vi "BinanceAPI_klinesParser.vi"(0 "String":string="[[1658347200000,\"23663.24000000\",\"23722.59000000\",\"23653.28000000\",\"23714.96000000\",\"256.13989000\",1658347379999,\"6067027.54690940\",9053,\"142.99676000\",\"3387101.46249020\",\"0\"],[1658347380000,\"23718.37000000\",\"23767.73000000\",\"23515.33000000\",\"23543.35000000\",\"946.67772000\",1658347559999,\"22402928.80379690\",22366,\"437.43972000\",\"10355818.28285050\",\"0\"],[1658347560000,\"23543.35000000\",\"23557.69000000\",\"23129.30000000\",\"23290.21000000\",\"3099.94602000\",1658347739999,\"72352782.71562150\",52417,\"1329.12545000\",\"30987661.71943290\",\"0\"],[1658347740000,\"23292.66000000\",\"23362.26000000\",\"23183.57000000\",\"23189.10000000\",\"1104.93990000\",1658347919999,\"25699483.56583190\",26655,\"548.60052000\",\"12760620.12435820\",\"0\"],[1658347920000,\"23186.61000000\",\"23227.93000000\",\"23080.00000000\",\"23085.06000000\",\"1535.74271000\",1658348099999,\"35542160.24309620\",31006,\"720.31062000\",\"16676896.47782450\",\"0\"],[1658348100000,\"23085.06000000\",\"23205.87000000\",\"23061.82000000\",\"23081.44000000\",\"1247.70886000\",1658348279999,\"28838715.14705330\",28358,\"589.19252000\",\"13619917.45208160\",\"0\"],[1658348280000,\"23081.44000000\",\"23146.70000000\",\"23002.89000000\",\"23124.56000000\",\"1176.89567000\",1658348459999,\"27140887.15973450\",27163,\"620.70218000\",\"14315259.40428540\",\"0\"],[1658348460000,\"23128.04000000\",\"23164.75000000\",\"22906.19000000\",\"23077.30000000\",\"2165.26684000\",1658348639999,\"49834566.81714380\",37258,\"1123.79793000\",\"25866736.24309830\",\"0\"],[1658348640000,\"23077.30000000\",\"23266.21000000\",\"23069.87000000\",\"23151.19000000\",\"1420.90968000\",1658348819999,\"32903334.24962870\",30888,\"652.00960000\",\"15098327.30678220\",\"0\"],[1658348820000,\"23154.51000000\",\"23193.68000000\",\"23000.61000000\",\"23030.72000000\",\"870.91964000\",1658348999999,\"20119457.31160460\",22367,\"423.83386000\",\"9792985.11733570\",\"0\"],[1658349000000,\"23030.28000000\",\"23123.57000000\",\"22969.29000000\",\"23104.71000000\",\"1005.49828000\",1658349179999,\"23177047.55477860\",22845,\"498.99542000\",\"11504775.92107370\",\"0\"],[1658349180000,\"23104.71000000\",\"23147.13000000\",\"23031.50000000\",\"23095.39000000\",\"536.59327000\",1658349359999,\"12392897.73165490\",14572,\"241.49870000\",\"5577724.99435290\",\"0\"],[1658349360000,\"23093.23000000\",\"23106.21000000\",\"23018.21000000\",\"23028.14000000\",\"458.30424000\",1658349539999,\"10572885.20125990\",12174,\"216.11603000\",\"4986224.12266900\",\"0\"],[1658349540000,\"23025.72000000\",\"23180.00000000\",\"23010.77000000\",\"23169.63000000\",\"730.04369000\",1658349719999,\"16865565.81021020\",17344,\"391.09889000\",\"9037203.89897580\",\"0\"],[1658349720000,\"23169.63000000\",\"23202.29000000\",\"23104.83000000\",\"23190.76000000\",\"518.70246000\",1658349899999,\"12018650.49457500\",14582,\"284.89408000\",\"6601983.75458750\",\"0\"],[1658349900000,\"23187.58000000\",\"23197.98000000\",\"23117.24000000\",\"23192.65000000\",\"423.00370000\",1658350079999,\"9793254.17683990\",12212,\"207.37017000\",\"4801293.50123250\",\"0\"],[1658350080000,\"23192.65000000\",\"23369.81000000\",\"23188.59000000\",\"23351.47000000\",\"1290.82207000\",1658350259999,\"30067083.65432220\",27695,\"723.29769000\",\"16848129.29270580\",\"0\"],[1658350260000,\"23351.47000000\",\"23370.00000000\",\"23301.63000000\",\"23329.33000000\",\"545.87360000\",1658350439999,\"12735271.72257250\",14658,\"273.13977000\",\"6373064.42542620\",\"0\"],[1658350440000,\"23325.07000000\",\"23348.17000000\",\"23246.78000000\",\"23290.83000000\",\"656.82732000\",1658350619999,\"15299488.59141300\",16542,\"316.26851000\",\"7366633.62180150\",\"0\"],[1658350620000,\"23286.79000000\",\"23315.69000000\",\"23219.44000000\",\"23259.70000000\",\"580.13747000\",1658350799999,\"13504072.32121060\",12670,\"227.22525000\",\"5291058.52408740\",\"0\"],[1658350800000,\"23262.32000000\",\"23307.25000000\",\"23252.06000000\",\"23273.16000000\",\"445.89775000\",1658350979999,\"10382095.07301540\",11907,\"237.41438000\",\"5527766.31736060\",\"0\"],[1658350980000,\"23273.16000000\",\"23317.35000000\",\"23238.07000000\",\"23292.57000000\",\"323.09746000\",1658351159999,\"7522267.57929260\",10583,\"164.20677000\",\"3823461.94073280\",\"0\"],[1658351160000,\"23295.15000000\",\"23408.75000000\",\"23290.50000000\",\"23403.41000000\",\"416.53763000\",1658351339999,\"9730537.88850020\",12557,\"246.43581000\",\"5757447.08477900\",\"0\"],[1658351340000,\"23400.59000000\",\"23404.35000000\",\"23347.74000000\",\"23350.85000000\",\"284.65292000\",1658351519999,\"6651358.99879110\",9465,\"156.28050000\",\"3651802.20196910\",\"0\"],[1658351520000,\"23350.85000000\",\"23388.66000000\",\"23306.08000000\",\"23380.89000000\",\"332.33084000\",1658351699999,\"7759502.79393790\",10066,\"164.48672000\",\"3840378.70951610\",\"0\"],[1658351700000,\"23383.71000000\",\"23389.00000000\",\"23322.20000000\",\"23330.09000000\",\"244.35332000\",1658351879999,\"5706758.02910410\",7878,\"114.35270000\",\"2670918.94295160\",\"0\"],[1658351880000,\"23330.09000000\",\"23382.27000000\",\"23326.32000000\",\"23378.93000000\",\"369.49055000\",1658352059999,\"8631353.96538760\",6569,\"114.80699000\",\"2681833.11026080\",\"0\"],[1658352060000,\"23380.36000000\",\"23434.00000000\",\"23340.00000000\",\"23372.76000000\",\"390.02511000\",1658352239999,\"9122737.93836740\",9832,\"194.24542000\",\"4543845.70816940\",\"0\"],[1658352240000,\"23372.76000000\",\"23372.77000000\",\"23287.28000000\",\"23312.51000000\",\"298.85056000\",1658352419999,\"6973644.48613640\",9193,\"144.27810000\",\"3367082.39989170\",\"0\"],[1658352420000,\"23312.51000000\",\"23345.51000000\",\"23299.38000000\",\"23340.11000000\",\"168.64549000\",1658352599999,\"3932176.69589520\",6031,\"97.74182000\",\"2279375.75222460\",\"0\"],[1658352600000,\"23340.11000000\",\"23347.26000000\",\"23266.42000000\",\"23295.75000000\",\"169.94898000\",1658352779999,\"3958141.00030790\",6143,\"71.57080000\",\"1666862.00138690\",\"0\"],[1658352780000,\"23297.61000000\",\"23350.00000000\",\"23277.48000000\",\"23347.10000000\",\"128.95247000\",1658352959999,\"3005102.45726760\",6498,\"70.34855000\",\"1639681.70112670\",\"0\"],[1658352960000,\"23347.60000000\",\"23379.99000000\",\"23343.23000000\",\"23345.48000000\",\"119.56860000\",1658353139999,\"2793086.41307330\",5469,\"65.88758000\",\"1539242.14634960\",\"0\"],[1658353140000,\"23345.48000000\",\"23347.41000000\",\"23319.58000000\",\"23334.83000000\",\"112.94594000\",1658353319999,\"2635310.06600650\",3781,\"70.77757000\",\"1651431.45277890\",\"0\"],[1658353320000,\"23334.83000000\",\"23700.00000000\",\"23334.83000000\",\"23665.41000000\",\"978.56393000\",1658353499999,\"23032794.93002870\",27892,\"584.67607000\",\"13755496.34479560\",\"0\"],[1658353500000,\"23665.41000000\",\"23799.62000000\",\"23581.75000000\",\"23768.58000000\",\"894.37276000\",1658353679999,\"21213256.93729260\",26896,\"441.60675000\",\"10477754.50332260\",\"0\"],[1658353680000,\"23768.58000000\",\"23769.61000000\",\"23574.81000000\",\"23725.45000000\",\"537.20727000\",1658353859999,\"12724890.73371940\",17629,\"289.57177000\",\"6860726.29343110\",\"0\"],[1658353860000,\"23725.45000000\",\"23733.39000000\",\"23648.88000000\",\"23665.25000000\",\"279.74513000\",1658354039999,\"6625353.22561640\",10688,\"117.34940000\",\"2779141.80989370\",\"0\"],[1658354040000,\"23665.78000000\",\"23686.37000000\",\"23623.54000000\",\"23643.00000000\",\"216.30745000\",1658354219999,\"5116543.37437430\",7874,\"101.28639000\",\"2395812.26952260\",\"0\"],[1658354220000,\"23643.57000000\",\"23652.78000000\",\"23584.36000000\",\"23608.15000000\",\"225.59837000\",1658354399999,\"5327858.79167780\",8462,\"84.56632000\",\"1997358.21979660\",\"0\"],[1658354400000,\"23607.06000000\",\"23616.03000000\",\"23526.38000000\",\"23563.66000000\",\"241.23563000\",1658354579999,\"5686089.41069430\",9460,\"116.03341000\",\"2735055.26742810\",\"0\"],[1658354580000,\"23563.66000000\",\"23641.78000000\",\"23530.04000000\",\"23591.30000000\",\"296.26889000\",1658354759999,\"6984079.86770860\",11005,\"155.97288000\",\"3676126.58231920\",\"0\"],[1658354760000,\"23591.30000000\",\"23635.05000000\",\"23570.20000000\",\"23600.29000000\",\"362.57920000\",1658354939999,\"8556514.96142100\",8070,\"279.40202000\",\"6593791.82218180\",\"0\"],[1658354940000,\"23601.05000000\",\"23601.13000000\",\"23550.00000000\",\"23558.75000000\",\"151.77531000\",1658355119999,\"3577751.06744300\",6127,\"67.94480000\",\"1601722.42267410\",\"0\"],[1658355120000,\"23557.75000000\",\"23579.22000000\",\"23475.00000000\",\"23485.09000000\",\"319.12747000\",1658355299999,\"7508488.55289070\",9656,\"113.02180000\",\"2659377.18639480\",\"0\"],[1658355300000,\"23486.61000000\",\"23544.30000000\",\"23438.76000000\",\"23532.51000000\",\"283.28390000\",1658355479999,\"6657018.16396230\",9873,\"157.38094000\",\"3698445.14656630\",\"0\"],[1658355480000,\"23532.51000000\",\"23538.92000000\",\"23485.02000000\",\"23526.25000000\",\"136.63635000\",1658355659999,\"3213734.04655520\",5849,\"67.83475000\",\"1595511.29869110\",\"0\"],[1658355660000,\"23525.46000000\",\"23581.51000000\",\"23523.52000000\",\"23575.73000000\",\"122.31247000\",1658355839999,\"2879548.45942340\",5190,\"78.42627000\",\"1846524.61665180\",\"0\"],[1658355840000,\"23573.40000000\",\"23584.32000000\",\"23535.77000000\",\"23537.14000000\",\"129.93788000\",1658356019999,\"3060488.05244040\",5764,\"68.74444000\",\"1619190.30047840\",\"0\"],[1658356020000,\"23537.14000000\",\"23550.00000000\",\"23495.01000000\",\"23532.31000000\",\"136.98964000\",1658356199999,\"3223035.76130240\",5999,\"61.78384000\",\"1453672.06304110\",\"0\"],[1658356200000,\"23532.31000000\",\"23574.10000000\",\"23531.00000000\",\"23532.76000000\",\"161.63923000\",1658356379999,\"3806461.12547130\",6658,\"82.11191000\",\"1933603.05814690\",\"0\"],[1658356380000,\"23532.76000000\",\"23533.52000000\",\"23412.99000000\",\"23469.88000000\",\"347.54851000\",1658356559999,\"8158857.45357220\",12563,\"149.67198000\",\"3513318.48321890\",\"0\"],[1658356560000,\"23468.16000000\",\"23492.70000000\",\"23355.00000000\",\"23449.50000000\",\"500.91394000\",1658356739999,\"11738707.50836680\",17277,\"224.26819000\",\"5256198.16761950\",\"0\"],[1658356740000,\"23449.50000000\",\"23460.02000000\",\"23383.93000000\",\"23417.79000000\",\"339.57720000\",1658356919999,\"7953168.25257930\",11805,\"156.70096000\",\"3670040.32626850\",\"0\"],[1658356920000,\"23417.79000000\",\"23445.23000000\",\"23401.59000000\",\"23430.62000000\",\"267.51977000\",1658357099999,\"6266283.00305560\",9666,\"140.04211000\",\"3280368.60094800\",\"0\"],[1658357100000,\"23429.11000000\",\"23430.62000000\",\"23360.00000000\",\"23370.05000000\",\"265.61983000\",1658357279999,\"6215299.54653220\",9837,\"111.43058000\",\"2607569.00195110\",\"0\"],[1658357280000,\"23367.17000000\",\"23410.00000000\",\"23353.04000000\",\"23358.65000000\",\"254.61880000\",1658357459999,\"5953358.79055690\",9842,\"118.64396000\",\"2774327.67614840\",\"0\"],[1658357460000,\"23358.65000000\",\"23376.13000000\",\"23310.43000000\",\"23314.33000000\",\"347.78864000\",1658357639999,\"8118965.53186380\",11790,\"167.28671000\",\"3905541.56132740\",\"0\"],[1658357640000,\"23314.33000000\",\"23367.51000000\",\"23314.33000000\",\"23334.57000000\",\"244.07032000\",1658357819999,\"5696893.81535380\",8896,\"142.33069000\",\"3322310.43938950\",\"0\"],[1658357820000,\"23337.11000000\",\"23357.02000000\",\"23304.56000000\",\"23309.06000000\",\"267.08519000\",1658357999999,\"6230380.52238170\",9247,\"138.65638000\",\"3234636.68335470\",\"0\"],[1658358000000,\"23309.06000000\",\"23334.71000000\",\"23256.69000000\",\"23267.98000000\",\"463.78513000\",1658358179999,\"10806427.81064560\",10604,\"171.91435000\",\"4006041.25282410\",\"0\"],[1658358180000,\"23267.98000000\",\"23280.04000000\",\"23184.25000000\",\"23208.48000000\",\"466.78368000\",1658358359999,\"10840482.69239380\",13918,\"218.86979000\",\"5083327.35367480\",\"0\"],[1658358360000,\"23211.61000000\",\"23300.21000000\",\"23206.00000000\",\"23289.09000000\",\"312.13044000\",1658358539999,\"7259768.03256200\",12194,\"170.57772000\",\"3967277.01586800\",\"0\"],[1658358540000,\"23288.05000000\",\"23317.55000000\",\"23245.00000000\",\"23250.16000000\",\"325.08373000\",1658358719999,\"7565935.03009150\",10181,\"175.10077000\",\"4075930.45346900\",\"0\"],[1658358720000,\"23250.16000000\",\"23265.73000000\",\"23203.57000000\",\"23229.81000000\",\"274.14894000\",1658358899999,\"6367956.05690610\",9199,\"120.91552000\",\"2808717.15305900\",\"0\"],[1658358900000,\"23231.96000000\",\"23264.93000000\",\"23142.57000000\",\"23166.74000000\",\"472.63810000\",1658359079999,\"10962667.84396380\",13410,\"218.02461000\",\"5057754.40926010\",\"0\"],[1658359080000,\"23166.74000000\",\"23231.73000000\",\"23111.00000000\",\"23206.58000000\",\"397.87286000\",1658359259999,\"9221050.64419060\",13655,\"213.01265000\",\"4937189.30769410\",\"0\"],[1658359260000,\"23206.58000000\",\"23268.70000000\",\"23183.30000000\",\"23258.90000000\",\"268.25098000\",1658359439999,\"6230138.32030960\",9875,\"140.72754000\",\"3268798.75356310\",\"0\"],[1658359440000,\"23258.90000000\",\"23287.07000000\",\"23196.00000000\",\"23226.58000000\",\"250.24962000\",1658359619999,\"5815762.30473550\",9116,\"134.23063000\",\"3120068.45655850\",\"0\"],[1658359620000,\"23226.58000000\",\"23244.98000000\",\"23194.14000000\",\"23222.75000000\",\"160.76538000\",1658359799999,\"3732929.12330670\",6448,\"74.87436000\",\"1738725.74384380\",\"0\"],[1658359800000,\"23220.19000000\",\"23251.54000000\",\"23212.84000000\",\"23244.42000000\",\"252.14758000\",1658359979999,\"5858987.19988250\",7956,\"139.04460000\",\"3231264.48457970\",\"0\"],[1658359980000,\"23244.42000000\",\"23357.16000000\",\"23242.73000000\",\"23324.83000000\",\"562.29606000\",1658360159999,\"13110606.53117060\",13800,\"332.75017000\",\"7759117.64943880\",\"0\"],[1658360160000,\"23324.83000000\",\"23347.65000000\",\"23281.71000000\",\"23344.22000000\",\"272.20599000\",1658360339999,\"6345444.66471060\",8282,\"129.69740000\",\"3023748.27259970\",\"0\"],[1658360340000,\"23344.22000000\",\"23391.38000000\",\"23324.61000000\",\"23357.36000000\",\"432.55840000\",1658360519999,\"10101989.86997870\",11211,\"259.52695000\",\"6061286.04227650\",\"0\"],[1658360520000,\"23357.36000000\",\"23396.00000000\",\"23334.43000000\",\"23369.18000000\",\"337.09891000\",1658360699999,\"7877032.48282710\",10322,\"180.01273000\",\"4206442.20913160\",\"0\"],[1658360700000,\"23366.76000000\",\"23401.88000000\",\"23350.00000000\",\"23359.99000000\",\"367.30987000\",1658360879999,\"8586184.09190920\",9435,\"164.34893000\",\"3842234.10386930\",\"0\"],[1658360880000,\"23359.99000000\",\"23378.43000000\",\"23291.13000000\",\"23317.11000000\",\"362.06150000\",1658361059999,\"8450662.03053600\",9310,\"148.28287000\",\"3460709.68962950\",\"0\"],[1658361060000,\"23317.11000000\",\"23326.40000000\",\"23200.44000000\",\"23203.93000000\",\"397.52029000\",1658361239999,\"9257249.64881010\",12151,\"178.48062000\",\"4157326.46055380\",\"0\"],[1658361240000,\"23204.74000000\",\"23268.19000000\",\"23183.10000000\",\"23212.22000000\",\"395.93654000\",1658361419999,\"9194436.55427420\",12573,\"187.68114000\",\"4358614.63933420\",\"0\"],[1658361420000,\"23209.65000000\",\"23241.10000000\",\"23174.67000000\",\"23223.30000000\",\"317.57370000\",1658361599999,\"7370760.20031100\",9690,\"157.06460000\",\"3645875.48688970\",\"0\"],[1658361600000,\"23223.30000000\",\"23280.21000000\",\"23200.00000000\",\"23261.54000000\",\"463.25824000\",1658361779999,\"10767488.43349340\",11878,\"239.67837000\",\"5571170.80147240\",\"0\"],[1658361780000,\"23259.78000000\",\"23314.18000000\",\"23218.01000000\",\"23304.48000000\",\"449.00293000\",1658361959999,\"10453936.81845270\",13318,\"240.94942000\",\"5609923.68490350\",\"0\"],[1658361960000,\"23303.20000000\",\"23317.78000000\",\"23253.39000000\",\"23297.83000000\",\"400.81855000\",1658362139999,\"9337284.98259050\",11991,\"198.82239000\",\"4631841.62327960\",\"0\"],[1658362140000,\"23297.83000000\",\"23315.61000000\",\"23263.93000000\",\"23313.50000000\",\"312.40358000\",1658362319999,\"7275388.40770780\",9482,\"170.74037000\",\"3976401.95753030\",\"0\"],[1658362320000,\"23315.61000000\",\"23350.00000000\",\"23263.66000000\",\"23318.27000000\",\"403.60469000\",1658362499999,\"9406760.13814050\",12022,\"203.22700000\",\"4736873.49560700\",\"0\"],[1658362500000,\"23320.68000000\",\"23386.55000000\",\"23307.91000000\",\"23383.39000000\",\"380.44823000\",1658362679999,\"8883227.63405430\",10580,\"233.56793000\",\"5454053.44543200\",\"0\"],[1658362680000,\"23385.53000000\",\"23386.56000000\",\"23324.21000000\",\"23336.46000000\",\"344.18601000\",1658362859999,\"8038148.69716000\",10173,\"154.85655000\",\"3616470.41552470\",\"0\"],[1658362860000,\"23337.43000000\",\"23339.57000000\",\"23271.40000000\",\"23309.54000000\",\"288.14946000\",1658363039999,\"6714350.49966780\",8922,\"139.56351000\",\"3252097.71397640\",\"0\"],[1658363040000,\"23306.75000000\",\"23334.47000000\",\"23305.02000000\",\"23321.45000000\",\"203.56761000\",1658363219999,\"4746665.90146060\",6832,\"104.78228000\",\"2443295.98027680\",\"0\"],[1658363220000,\"23320.76000000\",\"23348.88000000\",\"23263.24000000\",\"23275.65000000\",\"288.84692000\",1658363399999,\"6731525.37000290\",8880,\"142.81513000\",\"3328246.50960510\",\"0\"],[1658363400000,\"23275.65000000\",\"23282.09000000\",\"23219.72000000\",\"23247.51000000\",\"254.54668000\",1658363579999,\"5918363.44398710\",8334,\"130.64471000\",\"3037435.67776810\",\"0\"],[1658363580000,\"23250.45000000\",\"23254.13000000\",\"23125.00000000\",\"23148.05000000\",\"496.46138000\",1658363759999,\"11505300.14690320\",15124,\"201.66277000\",\"4672724.42245490\",\"0\"],[1658363760000,\"23148.36000000\",\"23221.19000000\",\"23142.00000000\",\"23205.00000000\",\"316.68401000\",1658363939999,\"7342108.47897450\",10074,\"181.63437000\",\"4211144.33656900\",\"0\"],[1658363940000,\"23204.30000000\",\"23206.08000000\",\"23164.95000000\",\"23186.24000000\",\"207.10079000\",1658364119999,\"4801088.55451220\",6923,\"97.75238000\",\"2266153.53402200\",\"0\"],[1658364120000,\"23185.56000000\",\"23200.00000000\",\"23143.15000000\",\"23156.40000000\",\"307.60396000\",1658364299999,\"7126756.39868770\",9282,\"148.03134000\",\"3429901.79666250\",\"0\"],[1658364300000,\"23156.40000000\",\"23191.36000000\",\"23122.34000000\",\"23127.11000000\",\"249.56613000\",1658364479999,\"5780614.14737820\",8355,\"119.76989000\",\"2774269.73107460\",\"0\"],[1658364480000,\"23127.11000000\",\"23175.29000000\",\"23124.65000000\",\"23157.72000000\",\"245.44872000\",1658364659999,\"5682647.90010750\",7937,\"118.12003000\",\"2734724.18187980\",\"0\"],[1658364660000,\"23157.72000000\",\"23211.56000000\",\"23150.02000000\",\"23202.50000000\",\"257.85819000\",1658364839999,\"5977052.10504890\",7840,\"143.23885000\",\"3320381.56935310\",\"0\"],[1658364840000,\"23204.25000000\",\"23267.00000000\",\"23184.43000000\",\"23258.73000000\",\"384.11208000\",1658365019999,\"8920740.54913490\",9756,\"266.40882000\",\"6187599.41639550\",\"0\"],[1658365020000,\"23261.20000000\",\"23276.81000000\",\"23229.28000000\",\"23249.70000000\",\"271.26077000\",1658365199999,\"6307356.11308370\",8670,\"165.52642000\",\"3849099.42916310\",\"0\"],[1658365200000,\"23249.70000000\",\"23312.40000000\",\"23233.07000000\",\"23276.78000000\",\"312.43249000\",1658365379999,\"7271846.46535520\",10029,\"163.17160000\",\"3797986.64275520\",\"0\"],[1658365380000,\"23276.78000000\",\"23302.68000000\",\"23249.67000000\",\"23259.14000000\",\"264.32372000\",1658365559999,\"6152576.59561360\",8370,\"120.86689000\",\"2813668.09538060\",\"0\"],[1658365560000,\"23257.00000000\",\"23294.55000000\",\"23255.42000000\",\"23272.47000000\",\"316.61138000\",1658365739999,\"7368051.92697860\",9505,\"170.44001000\",\"3966369.56429080\",\"0\"],[1658365740000,\"23272.47000000\",\"23289.00000000\",\"23228.95000000\",\"23274.51000000\",\"264.28432000\",1658365919999,\"6148749.23863140\",8936,\"122.00865000\",\"2838814.62197710\",\"0\"],[1658365920000,\"23271.63000000\",\"23442.77000000\",\"23271.63000000\",\"23387.75000000\",\"1133.04116000\",1658366099999,\"26480845.13176050\",27250,\"666.61993000\",\"15579337.89990070\",\"0\"],[1658366100000,\"23389.25000000\",\"23415.84000000\",\"23354.01000000\",\"23364.33000000\",\"372.78877000\",1658366279999,\"8717739.97083280\",12307,\"171.58377000\",\"4012615.56428620\",\"0\"],[1658366280000,\"23364.33000000\",\"23370.53000000\",\"23315.57000000\",\"23344.52000000\",\"304.04739000\",1658366459999,\"7096150.90589430\",10732,\"132.87540000\",\"3101342.08747430\",\"0\"],[1658366460000,\"23346.08000000\",\"23355.90000000\",\"23306.32000000\",\"23336.47000000\",\"260.54737000\",1658366639999,\"6080209.46876510\",8616,\"125.91385000\",\"2938632.88849920\",\"0\"],[1658366640000,\"23336.68000000\",\"23361.22000000\",\"23309.89000000\",\"23313.61000000\",\"206.50235000\",1658366819999,\"4820342.04657080\",7411,\"89.96991000\",\"2100230.98721260\",\"0\"],[1658366820000,\"23313.61000000\",\"23317.89000000\",\"23260.50000000\",\"23261.52000000\",\"275.89735000\",1658366999999,\"6426035.25033980\",9628,\"128.65356000\",\"2996806.27194320\",\"0\"],[1658367000000,\"23261.52000000\",\"23351.21000000\",\"23261.52000000\",\"23345.02000000\",\"345.41077000\",1658367179999,\"8051458.09266070\",9357,\"227.50385000\",\"5302830.05572770\",\"0\"],[1658367180000,\"23343.89000000\",\"23365.16000000\",\"23316.22000000\",\"23317.69000000\",\"223.37271000\",1658367359999,\"5213415.68472510\",7289,\"105.96245000\",\"2473242.49284200\",\"0\"],[1658367360000,\"23317.69000000\",\"23350.39000000\",\"23281.29000000\",\"23340.93000000\",\"308.81026000\",1658367539999,\"7201444.21662230\",7812,\"183.27437000\",\"4273642.49921770\",\"0\"],[1658367540000,\"23340.93000000\",\"23347.81000000\",\"23252.01000000\",\"23287.03000000\",\"297.67650000\",1658367719999,\"6936593.54656370\",9024,\"122.92064000\",\"2864489.34833310\",\"0\"],[1658367720000,\"23285.11000000\",\"23307.04000000\",\"23261.14000000\",\"23297.75000000\",\"176.90967000\",1658367899999,\"4119353.39839250\",6405,\"86.83037000\",\"2021908.85273900\",\"0\"],[1658367900000,\"23299.84000000\",\"23324.00000000\",\"23267.79000000\",\"23285.71000000\",\"227.65603000\",1658368079999,\"5303206.89868370\",7809,\"108.24133000\",\"2521635.12470070\",\"0\"],[1658368080000,\"23287.63000000\",\"23295.72000000\",\"23184.02000000\",\"23208.00000000\",\"520.08759000\",1658368259999,\"12083701.40575020\",12786,\"209.85647000\",\"4876419.35906320\",\"0\"],[1658368260000,\"23208.00000000\",\"23213.15000000\",\"23160.50000000\",\"23185.76000000\",\"350.10841000\",1658368439999,\"8117616.76381720\",11258,\"155.56243000\",\"3606910.48562090\",\"0\"],[1658368440000,\"23183.97000000\",\"23222.36000000\",\"23175.85000000\",\"23192.63000000\",\"217.72169000\",1658368619999,\"5051054.24211660\",6694,\"94.97356000\",\"2203196.80220310\",\"0\"],[1658368620000,\"23194.57000000\",\"23244.73000000\",\"23192.63000000\",\"23235.64000000\",\"180.14749000\",1658368799999,\"4184488.22910970\",5973,\"100.69159000\",\"2338889.82415860\",\"0\"],[1658368800000,\"23233.61000000\",\"23276.51000000\",\"23210.00000000\",\"23275.22000000\",\"201.79844000\",1658368979999,\"4689795.93140160\",6564,\"120.78505000\",\"2807199.10570030\",\"0\"],[1658368980000,\"23275.22000000\",\"23289.96000000\",\"23246.63000000\",\"23284.16000000\",\"245.80435000\",1658369159999,\"5719065.23896820\",8403,\"132.74859000\",\"3088721.22715620\",\"0\"],[1658369160000,\"23285.39000000\",\"23304.83000000\",\"23256.07000000\",\"23260.02000000\",\"210.15150000\",1658369339999,\"4892716.87108830\",7827,\"95.97449000\",\"2234504.66100190\",\"0\"],[1658369340000,\"23260.02000000\",\"23286.52000000\",\"23255.33000000\",\"23272.05000000\",\"152.98457000\",1658369519999,\"3560109.15038380\",6264,\"70.49879000\",\"1640579.52372330\",\"0\"],[1658369520000,\"23271.96000000\",\"23319.73000000\",\"23254.77000000\",\"23303.22000000\",\"177.96559000\",1658369699999,\"4144288.01238590\",7575,\"83.34037000\",\"1940741.68273900\",\"0\"],[1658369700000,\"23302.90000000\",\"23338.51000000\",\"23286.81000000\",\"23297.01000000\",\"214.67452000\",1658369879999,\"5003931.97197020\",8005,\"110.07523000\",\"2565984.71750630\",\"0\"],[1658369880000,\"23298.46000000\",\"23302.39000000\",\"23242.72000000\",\"23253.18000000\",\"200.96737000\",1658370059999,\"4679007.92376780\",7515,\"88.97316000\",\"2071763.38477320\",\"0\"],[1658370060000,\"23253.18000000\",\"23276.15000000\",\"23225.66000000\",\"23231.48000000\",\"178.49990000\",1658370239999,\"4150695.93534270\",7239,\"76.59734000\",\"1781115.64969440\",\"0\"],[1658370240000,\"23230.17000000\",\"23231.52000000\",\"23140.01000000\",\"23145.85000000\",\"561.05378000\",1658370419999,\"13000751.11893660\",15318,\"291.72524000\",\"6759551.68753480\",\"0\"],[1658370420000,\"23145.85000000\",\"23180.34000000\",\"23055.11000000\",\"23085.23000000\",\"650.70228000\",1658370599999,\"15043028.56485940\",15554,\"284.10873000\",\"6568534.39917380\",\"0\"],[1658370600000,\"23088.35000000\",\"23143.09000000\",\"23005.88000000\",\"23137.59000000\",\"888.86232000\",1658370779999,\"20504615.91328710\",20115,\"481.09116000\",\"11098485.83866730\",\"0\"],[1658370780000,\"23136.39000000\",\"23162.51000000\",\"23112.28000000\",\"23125.54000000\",\"286.18338000\",1658370959999,\"6620338.50898710\",8578,\"143.28294000\",\"3314840.00182330\",\"0\"],[1658370960000,\"23125.54000000\",\"23138.92000000\",\"23083.96000000\",\"23086.72000000\",\"210.75822000\",1658371139999,\"4869718.94849060\",7356,\"105.06350000\",\"2427752.43343720\",\"0\"],[1658371140000,\"23084.46000000\",\"23086.73000000\",\"23019.44000000\",\"23066.08000000\",\"591.14488000\",1658371319999,\"13622959.53228690\",16383,\"299.78492000\",\"6908849.76449340\",\"0\"],[1658371320000,\"23064.48000000\",\"23090.60000000\",\"22999.70000000\",\"23001.68000000\",\"668.87831000\",1658371499999,\"15403755.67917970\",14728,\"323.75699000\",\"7456581.31041900\",\"0\"],[1658371500000,\"23003.72000000\",\"23040.00000000\",\"22927.27000000\",\"22934.61000000\",\"959.67221000\",1658371679999,\"22046945.74246740\",22766,\"496.36822000\",\"11405255.13647860\",\"0\"],[1658371680000,\"22934.61000000\",\"22962.02000000\",\"22781.00000000\",\"22876.67000000\",\"1780.19341000\",1658371859999,\"40688265.37866640\",33726,\"730.34572000\",\"16698239.38875990\",\"0\"],[1658371860000,\"22876.67000000\",\"22877.88000000\",\"22809.07000000\",\"22812.90000000\",\"694.37998000\",1658372039999,\"15860142.65244200\",16933,\"358.13122000\",\"8180807.81419470\",\"0\"],[1658372040000,\"22810.08000000\",\"22860.00000000\",\"22714.32000000\",\"22750.41000000\",\"1197.58397000\",1658372219999,\"27271885.70606050\",25860,\"583.33603000\",\"13285722.68335050\",\"0\"],[1658372220000,\"22752.38000000\",\"22788.32000000\",\"22689.42000000\",\"22694.58000000\",\"870.62279000\",1658372399999,\"19784672.42809560\",20446,\"421.41391000\",\"9578329.13338610\",\"0\"],[1658372400000,\"22692.06000000\",\"22751.86000000\",\"22666.00000000\",\"22685.72000000\",\"877.96877000\",1658372579999,\"19937623.63091320\",19760,\"450.54340000\",\"10232467.57196810\",\"0\"],[1658372580000,\"22685.72000000\",\"22801.60000000\",\"22666.00000000\",\"22796.13000000\",\"613.42860000\",1658372759999,\"13957726.91317940\",16984,\"341.18701000\",\"7763524.48165710\",\"0\"],[1658372760000,\"22791.16000000\",\"22818.75000000\",\"22742.92000000\",\"22797.50000000\",\"404.15330000\",1658372939999,\"9207398.19913580\",12824,\"213.56735000\",\"4865813.64813140\",\"0\"],[1658372940000,\"22794.86000000\",\"22842.65000000\",\"22775.26000000\",\"22819.59000000\",\"446.11529000\",1658373119999,\"10178367.01236440\",11873,\"213.59517000\",\"4873371.68049190\",\"0\"],[1658373120000,\"22819.59000000\",\"22833.15000000\",\"22782.04000000\",\"22801.20000000\",\"334.79697000\",1658373299999,\"7635464.97150870\",9139,\"153.88983000\",\"3509856.73091830\",\"0\"],[1658373300000,\"22798.31000000\",\"22830.00000000\",\"22761.75000000\",\"22812.98000000\",\"409.48243000\",1658373479999,\"9338216.08893230\",10253,\"209.64773000\",\"4781706.93003050\",\"0\"],[1658373480000,\"22812.98000000\",\"22866.14000000\",\"22795.15000000\",\"22850.59000000\",\"350.30496000\",1658373659999,\"7999751.47456410\",10593,\"188.12841000\",\"4296239.75612310\",\"0\"],[1658373660000,\"22850.59000000\",\"22862.62000000\",\"22786.28000000\",\"22791.29000000\",\"306.14834000\",1658373839999,\"6985306.34180380\",9205,\"141.03058000\",\"3218032.32110630\",\"0\"],[1658373840000,\"22793.70000000\",\"22805.00000000\",\"22763.50000000\",\"22766.57000000\",\"312.65073000\",1658374019999,\"7124544.77328880\",8236,\"176.33995000\",\"4018827.86364920\",\"0\"],[1658374020000,\"22770.95000000\",\"22791.25000000\",\"22736.45000000\",\"22746.70000000\",\"367.39256000\",1658374199999,\"8363929.17098190\",9444,\"185.67806000\",\"4227495.66403850\",\"0\"],[1658374200000,\"22746.70000000\",\"22767.28000000\",\"22720.37000000\",\"22725.32000000\",\"320.52497000\",1658374379999,\"7291257.83408330\",9253,\"170.21626000\",\"3872145.41741460\",\"0\"],[1658374380000,\"22723.09000000\",\"22815.00000000\",\"22714.56000000\",\"22784.00000000\",\"438.25812000\",1658374559999,\"9979386.59112840\",11004,\"252.88486000\",\"5759396.75949850\",\"0\"],[1658374560000,\"22781.93000000\",\"22861.11000000\",\"22777.80000000\",\"22840.00000000\",\"368.61822000\",1658374739999,\"8414431.74217480\",10221,\"215.28027000\",\"4914252.37777180\",\"0\"],[1658374740000,\"22840.00000000\",\"22855.28000000\",\"22817.44000000\",\"22825.43000000\",\"193.02789000\",1658374919999,\"4407922.17692640\",6435,\"102.74168000\",\"2346405.53148700\",\"0\"],[1658374920000,\"22825.43000000\",\"22830.96000000\",\"22786.42000000\",\"22802.21000000\",\"195.88949000\",1658375099999,\"4467314.49293240\",6597,\"96.84888000\",\"2208671.68410580\",\"0\"],[1658375100000,\"22800.04000000\",\"22853.33000000\",\"22779.12000000\",\"22833.67000000\",\"273.14339000\",1658375279999,\"6231001.97816670\",8210,\"155.36255000\",\"3544333.69735580\",\"0\"],[1658375280000,\"22835.02000000\",\"22850.73000000\",\"22821.26000000\",\"22824.79000000\",\"217.42055000\",1658375459999,\"4964627.09314650\",6869,\"98.18174000\",\"2241989.32999280\",\"0\"],[1658375460000,\"22826.62000000\",\"22841.00000000\",\"22773.45000000\",\"22789.21000000\",\"265.77094000\",1658375639999,\"6061579.92042090\",7287,\"115.53074000\",\"2635091.45940750\",\"0\"],[1658375640000,\"22792.25000000\",\"22839.64000000\",\"22750.50000000\",\"22758.91000000\",\"443.64101000\",1658375819999,\"10110070.99845270\",10403,\"154.01525000\",\"3510513.26605280\",\"0\"],[1658375820000,\"22758.91000000\",\"22796.39000000\",\"22753.92000000\",\"22777.20000000\",\"180.43339000\",1658375999999,\"4109349.84048100\",6581,\"108.06550000\",\"2461206.78180420\",\"0\"],[1658376000000,\"22779.12000000\",\"22860.17000000\",\"22766.00000000\",\"22803.06000000\",\"624.08366000\",1658376179999,\"14242607.74976190\",12668,\"351.77477000\",\"8027617.19641070\",\"0\"],[1658376180000,\"22805.19000000\",\"22812.36000000\",\"22680.39000000\",\"22691.53000000\",\"851.87135000\",1658376359999,\"19381971.86382160\",15110,\"315.41776000\",\"7175318.71990640\",\"0\"],[1658376360000,\"22691.53000000\",\"22750.01000000\",\"22638.53000000\",\"22724.11000000\",\"1008.64261000\",1658376539999,\"22899759.35156330\",20452,\"464.01668000\",\"10534059.20509760\",\"0\"],[1658376540000,\"22723.78000000\",\"22787.50000000\",\"22690.46000000\",\"22751.59000000\",\"470.01808000\",1658376719999,\"10688383.26645950\",11750,\"252.13342000\",\"5733629.75660520\",\"0\"],[1658376720000,\"22751.59000000\",\"22763.17000000\",\"22718.20000000\",\"22755.20000000\",\"341.01248000\",1658376899999,\"7754338.08243520\",8484,\"208.08232000\",\"4731442.48223590\",\"0\"],[1658376900000,\"22750.61000000\",\"22802.41000000\",\"22746.03000000\",\"22794.96000000\",\"408.57760000\",1658377079999,\"9305641.44118390\",11170,\"223.92429000\",\"5100365.62645140\",\"0\"],[1658377080000,\"22794.96000000\",\"22802.77000000\",\"22776.60000000\",\"22794.88000000\",\"294.11685000\",1658377259999,\"6703134.18692500\",7395,\"156.70840000\",\"3571521.76969170\",\"0\"],[1658377260000,\"22794.83000000\",\"22795.56000000\",\"22755.78000000\",\"22756.52000000\",\"204.50335000\",1658377439999,\"4658589.01441900\",6234,\"92.06089000\",\"2097284.34299430\",\"0\"],[1658377440000,\"22760.53000000\",\"22772.69000000\",\"22712.38000000\",\"22733.18000000\",\"281.79796000\",1658377619999,\"6408382.31438280\",7348,\"135.75440000\",\"3087098.72860880\",\"0\"],[1658377620000,\"22733.18000000\",\"22777.04000000\",\"22700.08000000\",\"22732.43000000\",\"301.60760000\",1658377799999,\"6858667.67583850\",8048,\"158.66828000\",\"3608249.98051650\",\"0\"],[1658377800000,\"22734.00000000\",\"22831.08000000\",\"22717.69000000\",\"22814.74000000\",\"644.40953000\",1658377979999,\"14684176.73707260\",14268,\"371.97099000\",\"8476784.16623680\",\"0\"],[1658377980000,\"22814.74000000\",\"22833.35000000\",\"22789.05000000\",\"22822.29000000\",\"299.88180000\",1658378159999,\"6840748.13101670\",8427,\"150.74446000\",\"3439019.88347360\",\"0\"],[1658378160000,\"22823.99000000\",\"22829.17000000\",\"22797.31000000\",\"22822.18000000\",\"179.54466000\",1658378339999,\"4095678.11637340\",5161,\"98.79378000\",\"2253671.73509940\",\"0\"],[1658378340000,\"22822.18000000\",\"22878.00000000\",\"22811.02000000\",\"22840.39000000\",\"443.39911000\",1658378519999,\"10128517.47841070\",9604,\"225.29010000\",\"5146480.56808720\",\"0\"],[1658378520000,\"22840.39000000\",\"22888.00000000\",\"22830.47000000\",\"22858.37000000\",\"417.46955000\",1658378699999,\"9546413.51675720\",7883,\"161.31037000\",\"3688512.76331630\",\"0\"],[1658378700000,\"22858.37000000\",\"22892.89000000\",\"22856.13000000\",\"22888.38000000\",\"251.40187000\",1658378879999,\"5750248.72233290\",6526,\"136.62694000\",\"3125178.12108200\",\"0\"],[1658378880000,\"22888.38000000\",\"22935.20000000\",\"22881.86000000\",\"22918.86000000\",\"502.61385000\",1658379059999,\"11516825.09707570\",11687,\"223.62519000\",\"5124199.85448020\",\"0\"],[1658379060000,\"22917.73000000\",\"22943.18000000\",\"22896.59000000\",\"22896.64000000\",\"300.83256000\",1658379239999,\"6894034.50041330\",7761,\"186.66058000\",\"4277780.57181760\",\"0\"],[1658379240000,\"22899.10000000\",\"22931.50000000\",\"22885.69000000\",\"22912.37000000\",\"170.23739000\",1658379419999,\"3900599.29252590\",5955,\"97.66524000\",\"2237863.88990530\",\"0\"],[1658379420000,\"22912.37000000\",\"22918.95000000\",\"22866.18000000\",\"22881.41000000\",\"286.84166000\",1658379599999,\"6566875.72484430\",7709,\"140.80415000\",\"3223840.33303430\",\"0\"],[1658379600000,\"22881.41000000\",\"22913.10000000\",\"22869.29000000\",\"22899.87000000\",\"179.68967000\",1658379779999,\"4113095.50285550\",5836,\"97.40490000\",\"2229694.80322020\",\"0\"],[1658379780000,\"22899.87000000\",\"22922.00000000\",\"22896.44000000\",\"22917.21000000\",\"171.39995000\",1658379959999,\"3927027.64603680\",6162,\"99.29456000\",\"2275056.38301470\",\"0\"],[1658379960000,\"22917.21000000\",\"22930.43000000\",\"22910.64000000\",\"22929.14000000\",\"142.41097000\",1658380139999,\"3264355.08821520\",5214,\"74.34614000\",\"1704216.77589580\",\"0\"],[1658380140000,\"22929.14000000\",\"22936.67000000\",\"22920.00000000\",\"22931.62000000\",\"193.36071000\",1658380319999,\"4433527.71312080\",5576,\"75.83615000\",\"1738834.21112470\",\"0\"],[1658380320000,\"22931.62000000\",\"22935.32000000\",\"22882.50000000\",\"22903.79000000\",\"184.96537000\",1658380499999,\"4237120.58955230\",5724,\"90.72191000\",\"2078029.56335470\",\"0\"],[1658380500000,\"22903.79000000\",\"22928.04000000\",\"22886.35000000\",\"22917.26000000\",\"140.39499000\",1658380679999,\"3216149.91073640\",5374,\"76.50451000\",\"1752617.07443600\",\"0\"],[1658380680000,\"22918.77000000\",\"22968.46000000\",\"22915.00000000\",\"22943.43000000\",\"314.13101000\",1658380859999,\"7207616.19298830\",7972,\"204.50136000\",\"4692507.46622070\",\"0\"],[1658380860000,\"22943.43000000\",\"22946.09000000\",\"22920.03000000\",\"22931.99000000\",\"131.63220000\",1658381039999,\"3018445.48706260\",5073,\"70.98958000\",\"1627885.70138810\",\"0\"],[1658381040000,\"22929.25000000\",\"22934.46000000\",\"22899.86000000\",\"22906.08000000\",\"248.21723000\",1658381219999,\"5688907.53959740\",5981,\"96.33493000\",\"2207966.97046270\",\"0\"],[1658381220000,\"22903.57000000\",\"22927.03000000\",\"22880.00000000\",\"22885.18000000\",\"188.80546000\",1658381399999,\"4323476.09169620\",5794,\"93.86170000\",\"2149490.81723650\",\"0\"],[1658381400000,\"22885.18000000\",\"22896.28000000\",\"22839.94000000\",\"22847.38000000\",\"256.90405000\",1658381579999,\"5876608.11587860\",7009,\"99.90734000\",\"2285896.98827260\",\"0\"],[1658381580000,\"22847.38000000\",\"22867.23000000\",\"22828.46000000\",\"22855.98000000\",\"223.22515000\",1658381759999,\"5100693.42232280\",6565,\"116.60272000\",\"2664453.46352630\",\"0\"],[1658381760000,\"22857.64000000\",\"22858.18000000\",\"22813.27000000\",\"22845.60000000\",\"367.31704000\",1658381939999,\"8386322.37596330\",9281,\"178.19170000\",\"4068200.14336290\",\"0\"],[1658381940000,\"22842.72000000\",\"22993.71000000\",\"22840.08000000\",\"22951.81000000\",\"726.12788000\",1658382119999,\"16654888.53700440\",17175,\"412.53707000\",\"9461477.84328590\",\"0\"],[1658382120000,\"22951.81000000\",\"22951.81000000\",\"22909.72000000\",\"22918.92000000\",\"248.16104000\",1658382299999,\"5690251.63592150\",6888,\"112.98776000\",\"2590799.45426820\",\"0\"],[1658382300000,\"22918.92000000\",\"22944.30000000\",\"22868.60000000\",\"22893.38000000\",\"266.35280000\",1658382479999,\"6102652.38337950\",7519,\"115.33164000\",\"2642758.03614150\",\"0\"],[1658382480000,\"22896.03000000\",\"22934.36000000\",\"22874.45000000\",\"22925.18000000\",\"314.44447000\",1658382659999,\"7201154.69883880\",8012,\"171.79552000\",\"3934780.01653990\",\"0\"],[1658382660000,\"22922.55000000\",\"22977.07000000\",\"22920.00000000\",\"22954.99000000\",\"328.86120000\",1658382839999,\"7547801.20960840\",8661,\"186.44438000\",\"4279491.51163780\",\"0\"],[1658382840000,\"22954.99000000\",\"22967.31000000\",\"22866.63000000\",\"22909.93000000\",\"536.81207000\",1658383019999,\"12298087.69139920\",12500,\"223.16844000\",\"5112581.66185750\",\"0\"],[1658383020000,\"22907.31000000\",\"22945.63000000\",\"22891.87000000\",\"22942.00000000\",\"227.36534000\",1658383199999,\"5211381.78234630\",7506,\"114.70388000\",\"2629140.41163150\",\"0\"],[1658383200000,\"22943.15000000\",\"22948.65000000\",\"22916.24000000\",\"22922.55000000\",\"209.48163000\",1658383379999,\"4803746.93690640\",5994,\"108.92101000\",\"2497668.21469610\",\"0\"],[1658383380000,\"22920.43000000\",\"22937.78000000\",\"22904.68000000\",\"22924.56000000\",\"163.64493000\",1658383559999,\"3750758.09159140\",5979,\"82.04286000\",\"1880474.35091930\",\"0\"],[1658383560000,\"22926.67000000\",\"22964.67000000\",\"22911.38000000\",\"22946.26000000\",\"374.96605000\",1658383739999,\"8603558.27681430\",9379,\"212.27878000\",\"4870928.00449820\",\"0\"],[1658383740000,\"22946.26000000\",\"22967.57000000\",\"22937.70000000\",\"22942.59000000\",\"212.91666000\",1658383919999,\"4887115.27655360\",6503,\"100.48061000\",\"2306543.09886280\",\"0\"],[1658383920000,\"22940.22000000\",\"22963.24000000\",\"22939.00000000\",\"22953.57000000\",\"222.61792000\",1658384099999,\"5109407.86712630\",6435,\"125.43550000\",\"2879047.82131130\",\"0\"],[1658384100000,\"22953.57000000\",\"22953.57000000\",\"22917.05000000\",\"22923.07000000\",\"190.14514000\",1658384279999,\"4361832.81695020\",6526,\"86.46890000\",\"1983733.60690850\",\"0\"],[1658384280000,\"22923.07000000\",\"22944.37000000\",\"22903.43000000\",\"22928.21000000\",\"180.06834000\",1658384459999,\"4127660.43491110\",6245,\"79.72815000\",\"1827645.17770050\",\"0\"],[1658384460000,\"22931.45000000\",\"22938.72000000\",\"22885.19000000\",\"22908.28000000\",\"311.58441000\",1658384639999,\"7136634.70334500\",7953,\"170.22737000\",\"3898854.94508950\",\"0\"],[1658384640000,\"22905.78000000\",\"22928.91000000\",\"22890.73000000\",\"22915.26000000\",\"271.88054000\",1658384819999,\"6229485.56860730\",7448,\"162.10243000\",\"3714226.15544010\",\"0\"],[1658384820000,\"22916.57000000\",\"22936.83000000\",\"22876.01000000\",\"22882.69000000\",\"224.73649000\",1658384999999,\"5148892.23478750\",7214,\"109.87713000\",\"2518000.53228900\",\"0\"],[1658385000000,\"22882.69000000\",\"22890.00000000\",\"22806.25000000\",\"22826.61000000\",\"456.97170000\",1658385179999,\"10443029.49273590\",11939,\"198.20989000\",\"4529858.73189110\",\"0\"],[1658385180000,\"22829.04000000\",\"22857.36000000\",\"22823.41000000\",\"22842.99000000\",\"178.42730000\",1658385359999,\"4075677.74077730\",7071,\"94.23281000\",\"2152566.03852940\",\"0\"],[1658385360000,\"22840.82000000\",\"22882.37000000\",\"22840.82000000\",\"22864.71000000\",\"225.89921000\",1658385539999,\"5165389.69056830\",7561,\"120.05834000\",\"2745347.58441100\",\"0\"],[1658385540000,\"22864.70000000\",\"22873.92000000\",\"22831.72000000\",\"22863.53000000\",\"170.35168000\",1658385719999,\"3893056.08833230\",6540,\"81.69606000\",\"1866987.71892780\",\"0\"],[1658385720000,\"22863.53000000\",\"22877.58000000\",\"22845.84000000\",\"22857.81000000\",\"152.74665000\",1658385899999,\"3492018.47639480\",5967,\"74.32423000\",\"1699281.46230070\",\"0\"],[1658385900000,\"22857.81000000\",\"22862.83000000\",\"22813.33000000\",\"22819.50000000\",\"195.57316000\",1658386079999,\"4465692.00162510\",6596,\"85.61011000\",\"1954802.86704320\",\"0\"],[1658386080000,\"22819.50000000\",\"22827.08000000\",\"22750.14000000\",\"22804.05000000\",\"711.78081000\",1658386259999,\"16223086.43974410\",14767,\"327.02593000\",\"7454207.90476280\",\"0\"],[1658386260000,\"22798.75000000\",\"22811.70000000\",\"22755.13000000\",\"22801.04000000\",\"336.73897000\",1658386439999,\"7670544.43493360\",9670,\"155.25172000\",\"3536704.74040360\",\"0\"],[1658386440000,\"22803.11000000\",\"22833.14000000\",\"22793.10000000\",\"22822.63000000\",\"268.55820000\",1658386619999,\"6127836.89247470\",7636,\"156.47482000\",\"3570594.22088140\",\"0\"],[1658386620000,\"22822.63000000\",\"22824.85000000\",\"22773.07000000\",\"22790.23000000\",\"177.20604000\",1658386799999,\"4039364.91360110\",6753,\"63.01814000\",\"1436504.62145050\",\"0\"],[1658386800000,\"22790.23000000\",\"22812.05000000\",\"22773.49000000\",\"22812.02000000\",\"199.98118000\",1658386979999,\"4558446.91758840\",7111,\"97.40238000\",\"2220424.13180600\",\"0\"],[1658386980000,\"22812.02000000\",\"22827.27000000\",\"22778.27000000\",\"22796.92000000\",\"245.74473000\",1658387159999,\"5604657.15180260\",7543,\"121.33836000\",\"2767570.84143610\",\"0\"],[1658387160000,\"22796.90000000\",\"22874.27000000\",\"22781.97000000\",\"22865.26000000\",\"384.61423000\",1658387339999,\"8784370.57386480\",10206,\"229.90772000\",\"5251151.73593280\",\"0\"],[1658387340000,\"22865.26000000\",\"22921.12000000\",\"22843.50000000\",\"22904.99000000\",\"432.62601000\",1658387519999,\"9904425.33851090\",12614,\"245.86837000\",\"5628843.48165190\",\"0\"],[1658387520000,\"22904.99000000\",\"22943.94000000\",\"22882.51000000\",\"22912.64000000\",\"647.79025000\",1658387699999,\"14843731.20131320\",11463,\"290.60354000\",\"6659599.90530960\",\"0\"],[1658387700000,\"22912.64000000\",\"22943.21000000\",\"22865.55000000\",\"22941.54000000\",\"420.55435000\",1658387879999,\"9631843.50574210\",9617,\"233.31441000\",\"5343540.28151000\",\"0\"],[1658387880000,\"22936.96000000\",\"23099.51000000\",\"22932.96000000\",\"23057.10000000\",\"1739.25815000\",1658388059999,\"40057271.17942390\",26386,\"741.81748000\",\"17084765.79160620\",\"0\"],[1658388060000,\"23057.10000000\",\"23082.60000000\",\"23047.35000000\",\"23049.03000000\",\"355.88216000\",1658388239999,\"8206660.37207080\",9719,\"167.53008000\",\"3863488.74113670\",\"0\"],[1658388240000,\"23047.36000000\",\"23050.96000000\",\"22955.52000000\",\"23010.00000000\",\"499.60329000\",1658388419999,\"11490645.33288960\",13045,\"233.08045000\",\"5360555.84677680\",\"0\"],[1658388420000,\"23010.00000000\",\"23019.81000000\",\"22983.81000000\",\"22998.08000000\",\"200.72656000\",1658388599999,\"4616885.16137110\",7703,\"102.69488000\",\"2362114.45552810\",\"0\"],[1658388600000,\"22998.08000000\",\"23006.75000000\",\"22956.01000000\",\"22973.79000000\",\"217.33793000\",1658388779999,\"4994168.82331690\",7408,\"111.10109000\",\"2553121.14735140\",\"0\"],[1658388780000,\"22973.79000000\",\"22975.68000000\",\"22940.70000000\",\"22941.03000000\",\"261.64217000\",1658388959999,\"6006671.09483550\",7636,\"96.01176000\",\"2204397.80781890\",\"0\"],[1658388960000,\"22944.12000000\",\"23032.23000000\",\"22928.89000000\",\"23022.21000000\",\"381.25189000\",1658389139999,\"8763041.15805490\",10219,\"202.68765000\",\"4658429.65086230\",\"0\"],[1658389140000,\"23022.21000000\",\"23038.44000000\",\"22980.32000000\",\"22993.68000000\",\"266.72718000\",1658389319999,\"6137314.14042570\",8125,\"120.02034000\",\"2761803.80804330\",\"0\"],[1658389320000,\"22993.69000000\",\"23009.91000000\",\"22966.45000000\",\"22989.99000000\",\"241.70446000\",1658389499999,\"5555191.41622610\",7983,\"114.38061000\",\"2628989.62966860\",\"0\"],[1658389500000,\"22989.99000000\",\"23000.00000000\",\"22973.18000000\",\"22976.65000000\",\"158.39607000\",1658389679999,\"3641235.53285830\",6618,\"74.57911000\",\"1714508.07042070\",\"0\"],[1658389680000,\"22978.75000000\",\"22981.87000000\",\"22938.99000000\",\"22947.42000000\",\"219.12320000\",1658389859999,\"5030866.76187350\",7463,\"102.22774000\",\"2347137.76131960\",\"0\"],[1658389860000,\"22949.51000000\",\"22980.09000000\",\"22920.80000000\",\"22970.73000000\",\"253.56143000\",1658390039999,\"5819190.95566990\",8112,\"130.43720000\",\"2993625.69932110\",\"0\"],[1658390040000,\"22970.73000000\",\"22979.55000000\",\"22955.14000000\",\"22962.05000000\",\"257.47149000\",1658390219999,\"5913804.16505150\",6850,\"121.06409000\",\"2780632.07660740\",\"0\"],[1658390220000,\"22962.05000000\",\"22964.33000000\",\"22919.33000000\",\"22931.56000000\",\"217.43307000\",1658390399999,\"4987771.82405600\",7121,\"98.72213000\",\"2264794.84287690\",\"0\"],[1658390400000,\"22929.28000000\",\"22936.26000000\",\"22880.50000000\",\"22921.29000000\",\"427.53097000\",1658390579999,\"9792635.79032000\",11315,\"188.51373000\",\"4317950.35628020\",\"0\"],[1658390580000,\"22921.29000000\",\"22971.34000000\",\"22910.00000000\",\"22935.80000000\",\"279.66069000\",1658390759999,\"6415552.01937990\",8685,\"154.73621000\",\"3549956.43260070\",\"0\"],[1658390760000,\"22935.80000000\",\"22939.07000000\",\"22900.00000000\",\"22926.48000000\",\"301.24596000\",1658390939999,\"6903706.34004860\",8825,\"147.43593000\",\"3379202.07618100\",\"0\"],[1658390940000,\"22926.48000000\",\"22934.48000000\",\"22910.42000000\",\"22928.89000000\",\"129.96802000\",1658391119999,\"2979205.29757110\",5528,\"66.83450000\",\"1532063.22619490\",\"0\"],[1658391120000,\"22928.90000000\",\"22931.53000000\",\"22872.50000000\",\"22886.16000000\",\"267.39027000\",1658391299999,\"6123609.48497560\",7855,\"113.77128000\",\"2605609.65347740\",\"0\"],[1658391300000,\"22886.16000000\",\"22932.09000000\",\"22863.78000000\",\"22924.16000000\",\"279.66147000\",1658391479999,\"6404613.75773770\",8916,\"153.49100000\",\"3515508.74294250\",\"0\"],[1658391480000,\"22922.19000000\",\"22924.35000000\",\"22850.69000000\",\"22853.60000000\",\"215.96850000\",1658391659999,\"4941549.48785070\",7271,\"91.79903000\",\"2100462.39088830\",\"0\"],[1658391660000,\"22853.60000000\",\"22888.84000000\",\"22837.92000000\",\"22851.63000000\",\"292.77461000\",1658391839999,\"6694424.51584300\",8748,\"142.01439000\",\"3247375.07608080\",\"0\"],[1658391840000,\"22851.63000000\",\"22859.00000000\",\"22815.86000000\",\"22837.55000000\",\"309.40893000\",1658392019999,\"7066768.10339130\",9894,\"155.39354000\",\"3549220.35745520\",\"0\"],[1658392020000,\"22838.72000000\",\"22851.82000000\",\"22820.00000000\",\"22835.28000000\",\"174.51439000\",1658392199999,\"3985382.35038390\",6620,\"88.78070000\",\"2027502.90973130\",\"0\"],[1658392200000,\"22833.56000000\",\"22859.99000000\",\"22820.69000000\",\"22856.91000000\",\"192.83593000\",1658392379999,\"4404868.03625510\",7521,\"100.41024000\",\"2293751.77845230\",\"0\"],[1658392380000,\"22856.91000000\",\"22911.16000000\",\"22851.37000000\",\"22868.92000000\",\"324.03507000\",1658392559999,\"7415448.31160220\",9537,\"178.53841000\",\"4085879.73469440\",\"0\"],[1658392560000,\"22867.24000000\",\"22904.87000000\",\"22863.57000000\",\"22893.04000000\",\"241.48843000\",1658392739999,\"5526402.51428680\",7267,\"128.86156000\",\"2948990.57325590\",\"0\"],[1658392740000,\"22895.25000000\",\"22915.22000000\",\"22836.68000000\",\"22873.35000000\",\"556.71895000\",1658392919999,\"12741179.16748020\",12205,\"321.48285000\",\"7359135.44422970\",\"0\"],[1658392920000,\"22875.80000000\",\"22887.78000000\",\"22825.91000000\",\"22829.94000000\",\"555.99498000\",1658393099999,\"12708125.11815770\",14191,\"281.89757000\",\"6443831.51286480\",\"0\"],[1658393100000,\"22833.37000000\",\"22842.10000000\",\"22797.03000000\",\"22810.73000000\",\"432.04330000\",1658393279999,\"9857324.55330810\",10049,\"227.04479000\",\"5180439.81705170\",\"0\"],[1658393280000,\"22808.69000000\",\"22881.12000000\",\"22800.27000000\",\"22873.77000000\",\"312.45927000\",1658393459999,\"7133303.77650850\",9083,\"204.71151000\",\"4673806.81971470\",\"0\"],[1658393460000,\"22873.45000000\",\"22897.22000000\",\"22842.81000000\",\"22857.82000000\",\"267.54929000\",1658393639999,\"6117809.95680980\",8423,\"138.13486000\",\"3158797.77054820\",\"0\"],[1658393640000,\"22856.28000000\",\"22870.65000000\",\"22844.45000000\",\"22859.55000000\",\"157.54947000\",1658393819999,\"3601280.40439370\",5903,\"91.83657000\",\"2099290.10136510\",\"0\"],[1658393820000,\"22862.30000000\",\"22878.77000000\",\"22851.70000000\",\"22878.77000000\",\"146.64888000\",1658393999999,\"3352970.57750520\",5933,\"75.89196000\",\"1735258.96881760\",\"0\"],[1658394000000,\"22878.77000000\",\"22887.76000000\",\"22866.20000000\",\"22883.54000000\",\"152.31468000\",1658394179999,\"3484506.62602830\",6021,\"75.83327000\",\"1734935.32494880\",\"0\"],[1658394180000,\"22883.54000000\",\"22889.06000000\",\"22855.29000000\",\"22887.27000000\",\"228.85878000\",1658394359999,\"5233703.64289330\",7194,\"115.38850000\",\"2639020.63786090\",\"0\"],[1658394360000,\"22886.79000000\",\"22951.97000000\",\"22884.10000000\",\"22893.30000000\",\"499.62268000\",1658394539999,\"11448770.93012090\",11873,\"298.63996000\",\"6843206.11955470\",\"0\"],[1658394540000,\"22891.35000000\",\"22935.77000000\",\"22891.33000000\",\"22928.55000000\",\"218.25781000\",1658394719999,\"5000495.67707020\",7276,\"118.05086000\",\"2704672.92922560\",\"0\"],[1658394720000,\"22927.40000000\",\"22970.90000000\",\"22916.74000000\",\"22948.39000000\",\"402.35551000\",1658394899999,\"9230663.78449500\",11148,\"204.94155000\",\"4701610.74035630\",\"0\"],[1658394900000,\"22949.66000000\",\"23002.63000000\",\"22943.91000000\",\"22990.57000000\",\"502.21338000\",1658395079999,\"11539081.45203720\",13482,\"257.41829000\",\"5915119.23715040\",\"0\"],[1658395080000,\"22987.48000000\",\"23004.31000000\",\"22964.40000000\",\"22997.24000000\",\"374.15279000\",1658395259999,\"8601305.04050000\",10843,\"204.00695000\",\"4690005.52921410\",\"0\"],[1658395260000,\"22994.94000000\",\"22997.28000000\",\"22930.61000000\",\"22940.46000000\",\"261.57552000\",1658395439999,\"6006450.16647190\",8785,\"109.30566000\",\"2510125.09450610\",\"0\"],[1658395440000,\"22940.46000000\",\"22984.09000000\",\"22916.83000000\",\"22974.95000000\",\"366.11048000\",1658395619999,\"8403427.60175220\",9505,\"184.88870000\",\"4243870.26641410\",\"0\"],[1658395620000,\"22971.76000000\",\"22978.35000000\",\"22935.55000000\",\"22947.37000000\",\"221.41411000\",1658395799999,\"5082528.90967880\",7661,\"103.93921000\",\"2385915.18790580\",\"0\"],[1658395800000,\"22947.37000000\",\"23000.00000000\",\"22934.91000000\",\"22992.48000000\",\"211.43008000\",1658395979999,\"4855278.42314780\",7010,\"126.79597000\",\"2912173.18897860\",\"0\"],[1658395980000,\"22990.95000000\",\"23022.54000000\",\"22945.66000000\",\"22947.25000000\",\"328.36529000\",1658396159999,\"7546839.94344890\",9083,\"171.51209000\",\"3942078.19359990\",\"0\"],[1658396160000,\"22949.61000000\",\"22970.98000000\",\"22942.00000000\",\"22961.32000000\",\"143.57179000\",1658396339999,\"3295516.08117440\",5702,\"83.47467000\",\"1916102.48350980\",\"0\"],[1658396340000,\"22961.32000000\",\"22974.27000000\",\"22924.17000000\",\"22960.58000000\",\"252.86384000\",1658396519999,\"5803525.99576260\",7641,\"119.41055000\",\"2740689.79252690\",\"0\"],[1658396520000,\"22963.46000000\",\"22983.89000000\",\"22945.31000000\",\"22950.70000000\",\"221.04601000\",1658396699999,\"5076082.30296960\",7428,\"105.86488000\",\"2431165.73387100\",\"0\"],[1658396700000,\"22950.70000000\",\"22988.00000000\",\"22944.53000000\",\"22980.77000000\",\"214.31536000\",1658396879999,\"4921547.76552000\",7323,\"118.90269000\",\"2730772.03082620\",\"0\"],[1658396880000,\"22983.53000000\",\"22993.64000000\",\"22940.63000000\",\"22945.62000000\",\"236.55521000\",1658397059999,\"5432924.00784820\",8017,\"111.95963000\",\"2571691.49717520\",\"0\"],[1658397060000,\"22945.62000000\",\"22986.52000000\",\"22928.48000000\",\"22972.28000000\",\"298.47844000\",1658397239999,\"6853351.74839070\",8938,\"179.47309000\",\"4120922.14224560\",\"0\"],[1658397240000,\"22970.11000000\",\"22998.00000000\",\"22958.86000000\",\"22986.30000000\",\"246.73385000\",1658397419999,\"5670591.85571780\",8201,\"125.94080000\",\"2894674.99177830\",\"0\"],[1658397420000,\"22986.30000000\",\"23006.57000000\",\"22971.46000000\",\"23003.58000000\",\"205.86029000\",1658397599999,\"4732907.98005690\",7145,\"125.24913000\",\"2879701.68286560\",\"0\"],[1658397600000,\"23003.58000000\",\"23039.67000000\",\"22979.54000000\",\"23032.52000000\",\"399.34853000\",1658397779999,\"9186461.90802340\",11132,\"240.64782000\",\"5536038.50434450\",\"0\"],[1658397780000,\"23034.26000000\",\"23057.78000000\",\"23005.39000000\",\"23023.34000000\",\"316.96058000\",1658397959999,\"7299589.92089620\",10716,\"175.71287000\",\"4046778.99419850\",\"0\"],[1658397960000,\"23025.60000000\",\"23031.91000000\",\"23002.95000000\",\"23027.49000000\",\"232.17639000\",1658398139999,\"5343852.42254820\",7990,\"110.62503000\",\"2546269.29116590\",\"0\"],[1658398140000,\"23024.59000000\",\"23048.87000000\",\"22996.98000000\",\"23026.53000000\",\"350.87691000\",1658398319999,\"8078056.76425320\",9317,\"141.78906000\",\"3264505.58554490\",\"0\"],[1658398320000,\"23026.54000000\",\"23074.12000000\",\"23019.00000000\",\"23050.27000000\",\"260.36195000\",1658398499999,\"5998875.14884080\",8560,\"143.98826000\",\"3317708.51668410\",\"0\"],[1658398500000,\"23050.27000000\",\"23071.44000000\",\"23008.01000000\",\"23013.57000000\",\"278.31312000\",1658398679999,\"6412434.98167830\",9317,\"142.63446000\",\"3286538.17011550\",\"0\"],[1658398680000,\"23013.57000000\",\"23016.17000000\",\"22972.24000000\",\"23005.04000000\",\"316.86137000\",1658398859999,\"7286940.15762550\",9315,\"173.75114000\",\"3995906.65356120\",\"0\"],[1658398860000,\"23005.04000000\",\"23007.58000000\",\"22974.98000000\",\"22993.41000000\",\"305.31864000\",1658399039999,\"7018576.34409120\",8529,\"141.34760000\",\"3249325.71200520\",\"0\"],[1658399040000,\"22993.41000000\",\"22999.48000000\",\"22966.32000000\",\"22977.85000000\",\"231.80601000\",1658399219999,\"5327001.49873450\",7498,\"95.84516000\",\"2202670.72371250\",\"0\"],[1658399220000,\"22977.85000000\",\"22985.76000000\",\"22958.37000000\",\"22972.31000000\",\"178.20296000\",1658399399999,\"4093841.47361100\",6633,\"87.44139000\",\"2008956.47039280\",\"0\"],[1658399400000,\"22970.34000000\",\"23000.59000000\",\"22958.01000000\",\"22973.49000000\",\"268.10925000\",1658399579999,\"6161946.16535390\",9132,\"128.93400000\",\"2963458.27059010\",\"0\"],[1658399580000,\"22971.69000000\",\"22977.00000000\",\"22937.02000000\",\"22950.84000000\",\"228.20147000\",1658399759999,\"5237842.66226200\",7988,\"115.37167000\",\"2648166.35437760\",\"0\"],[1658399760000,\"22950.84000000\",\"22959.90000000\",\"22937.41000000\",\"22953.28000000\",\"184.15400000\",1658399939999,\"4226081.25687060\",7045,\"94.75421000\",\"2174566.27188540\",\"0\"],[1658399940000,\"22955.00000000\",\"22964.12000000\",\"22931.00000000\",\"22947.19000000\",\"271.76044000\",1658400119999,\"6236145.26080700\",8142,\"145.48737000\",\"3338686.69213890\",\"0\"],[1658400120000,\"22947.19000000\",\"22954.66000000\",\"22935.00000000\",\"22945.87000000\",\"220.00989000\",1658400299999,\"5047614.25447990\",7025,\"155.88410000\",\"3576457.12111180\",\"0\"],[1658400300000,\"22945.87000000\",\"22954.45000000\",\"22935.78000000\",\"22939.96000000\",\"166.28591000\",1658400479999,\"3815242.09580000\",6684,\"92.28674000\",\"2117446.23542700\",\"0\"],[1658400480000,\"22941.63000000\",\"22960.62000000\",\"22923.59000000\",\"22943.63000000\",\"208.85245000\",1658400659999,\"4791443.50315880\",8540,\"108.52271000\",\"2489719.12608130\",\"0\"],[1658400660000,\"22946.87000000\",\"22980.09000000\",\"22943.63000000\",\"22952.72000000\",\"194.65942000\",1658400839999,\"4470091.35245520\",7535,\"113.62805000\",\"2609383.67815740\",\"0\"],[1658400840000,\"22952.72000000\",\"22954.73000000\",\"22885.00000000\",\"22902.38000000\",\"440.25432000\",1658401019999,\"10084490.83086460\",11569,\"189.94875000\",\"4350871.59529620\",\"0\"],[1658401020000,\"22904.29000000\",\"22908.06000000\",\"22846.95000000\",\"22869.55000000\",\"359.42875000\",1658401199999,\"8222398.69070540\",10032,\"182.31364000\",\"4170603.41238790\",\"0\"],[1658401200000,\"22870.88000000\",\"22878.33000000\",\"22827.58000000\",\"22832.19000000\",\"311.53208000\",1658401379999,\"7118412.72356050\",9464,\"152.06684000\",\"3474937.57620450\",\"0\"],[1658401380000,\"22832.19000000\",\"22865.56000000\",\"22817.93000000\",\"22852.60000000\",\"369.88390000\",1658401559999,\"8448846.39341650\",11027,\"201.78029000\",\"4609285.61970110\",\"0\"],[1658401560000,\"22852.60000000\",\"22888.00000000\",\"22844.72000000\",\"22881.37000000\",\"217.73664000\",1658401739999,\"4978640.66978540\",7830,\"129.78175000\",\"2967612.17040220\",\"0\"],[1658401740000,\"22881.37000000\",\"22906.87000000\",\"22850.63000000\",\"22850.63000000\",\"302.81163000\",1658401919999,\"6929118.61308830\",8806,\"145.34593000\",\"3326500.99181780\",\"0\"],[1658401920000,\"22853.61000000\",\"22853.62000000\",\"22662.65000000\",\"22699.53000000\",\"1046.41872000\",1658402099999,\"23822679.26519460\",20970,\"395.48112000\",\"9002703.85722050\",\"0\"],[1658402100000,\"22698.21000000\",\"22740.00000000\",\"22650.00000000\",\"22716.47000000\",\"860.01313000\",1658402279999,\"19519878.53062770\",21303,\"460.84065000\",\"10461840.19543610\",\"0\"],[1658402280000,\"22718.42000000\",\"22778.90000000\",\"22708.04000000\",\"22724.75000000\",\"703.91157000\",1658402459999,\"16009241.59192930\",14252,\"431.45165000\",\"9813188.07878430\",\"0\"],[1658402460000,\"22722.03000000\",\"22795.00000000\",\"22722.03000000\",\"22746.10000000\",\"476.50023000\",1658402639999,\"10843738.75501340\",10497,\"285.83867000\",\"6505353.96856580\",\"0\"],[1658402640000,\"22742.85000000\",\"22748.58000000\",\"22692.62000000\",\"22708.75000000\",\"450.22786000\",1658402819999,\"10227580.72239830\",10140,\"245.28853000\",\"5571985.15440420\",\"0\"],[1658402820000,\"22708.91000000\",\"22730.62000000\",\"22466.34000000\",\"22562.44000000\",\"1976.24407000\",1658402999999,\"44583666.16286020\",34168,\"856.17116000\",\"19311062.30014440\",\"0\"],[1658403000000,\"22562.44000000\",\"22637.26000000\",\"22536.34000000\",\"22597.25000000\",\"868.43448000\",1658403179999,\"19622764.45435830\",18482,\"467.79452000\",\"10569862.96765350\",\"0\"],[1658403180000,\"22594.52000000\",\"22647.74000000\",\"22570.14000000\",\"22632.26000000\",\"1194.97140000\",1658403359999,\"27011441.13157010\",21445,\"810.34086000\",\"18316918.09918060\",\"0\"],[1658403360000,\"22633.74000000\",\"22636.69000000\",\"22555.57000000\",\"22593.70000000\",\"705.06683000\",1658403539999,\"15925659.39825940\",16742,\"358.19987000\",\"8091310.93737440\",\"0\"],[1658403540000,\"22593.50000000\",\"22598.86000000\",\"22540.65000000\",\"22554.47000000\",\"512.40950000\",1658403719999,\"11562297.22239780\",13948,\"256.05004000\",\"5778032.22542090\",\"0\"],[1658403720000,\"22554.47000000\",\"22611.99000000\",\"22551.24000000\",\"22606.38000000\",\"456.56067000\",1658403899999,\"10312507.04765190\",12420,\"259.53849000\",\"5862714.99864330\",\"0\"],[1658403900000,\"22609.62000000\",\"22664.03000000\",\"22590.02000000\",\"22625.69000000\",\"579.11977000\",1658404079999,\"13106692.85888270\",11796,\"303.91456000\",\"6878854.41662260\",\"0\"],[1658404080000,\"22623.97000000\",\"22663.64000000\",\"22617.00000000\",\"22657.13000000\",\"378.06206000\",1658404259999,\"8562473.84216890\",8461,\"169.43015000\",\"3837433.83433870\",\"0\"],[1658404260000,\"22654.89000000\",\"22657.13000000\",\"22610.02000000\",\"22619.50000000\",\"263.41905000\",1658404439999,\"5962299.66722590\",7573,\"119.31879000\",\"2700839.09897020\",\"0\"],[1658404440000,\"22620.35000000\",\"22623.02000000\",\"22580.78000000\",\"22595.20000000\",\"386.00180000\",1658404619999,\"8724068.43833840\",8670,\"207.45762000\",\"4688988.15731560\",\"0\"],[1658404620000,\"22593.14000000\",\"22634.00000000\",\"22591.00000000\",\"22606.04000000\",\"281.83623000\",1658404799999,\"6372090.74151090\",7682,\"149.76152000\",\"3386060.48105930\",\"0\"],[1658404800000,\"22607.92000000\",\"22656.67000000\",\"22574.77000000\",\"22641.23000000\",\"500.03076000\",1658404979999,\"11304246.86517680\",10091,\"232.72517000\",\"5262242.76223790\",\"0\"],[1658404980000,\"22641.23000000\",\"22650.00000000\",\"22565.78000000\",\"22572.07000000\",\"426.74300000\",1658405159999,\"9645393.00615060\",10290,\"150.66732000\",\"3405873.31804750\",\"0\"],[1658405160000,\"22569.15000000\",\"22662.28000000\",\"22542.14000000\",\"22615.72000000\",\"589.96260000\",1658405339999,\"13332466.38648180\",13302,\"287.87047000\",\"6506559.26027990\",\"0\"],[1658405340000,\"22612.61000000\",\"22685.88000000\",\"22596.35000000\",\"22681.06000000\",\"565.58847000\",1658405519999,\"12813855.68735770\",12781,\"329.29847000\",\"7461105.08083700\",\"0\"],[1658405520000,\"22681.06000000\",\"22703.66000000\",\"22652.10000000\",\"22662.53000000\",\"319.72225000\",1658405699999,\"7250387.72067070\",10663,\"165.62433000\",\"3756203.15783280\",\"0\"],[1658405700000,\"22662.53000000\",\"22669.42000000\",\"22585.35000000\",\"22637.37000000\",\"900.49379000\",1658405879999,\"20373870.87933170\",19295,\"462.42336000\",\"10462421.56854710\",\"0\"],[1658405880000,\"22634.55000000\",\"22754.19000000\",\"22628.44000000\",\"22745.80000000\",\"745.25857000\",1658406059999,\"16918082.82572770\",16954,\"395.47784000\",\"8977868.46905820\",\"0\"],[1658406060000,\"22742.71000000\",\"22783.19000000\",\"22730.22000000\",\"22761.70000000\",\"595.50388000\",1658406239999,\"13548733.71707160\",13224,\"326.54768000\",\"7430004.44116210\",\"0\"],[1658406240000,\"22761.70000000\",\"22768.95000000\",\"22706.04000000\",\"22736.18000000\",\"414.58761000\",1658406419999,\"9424837.63369940\",11264,\"200.64429000\",\"4561133.88255320\",\"0\"],[1658406420000,\"22736.18000000\",\"22759.30000000\",\"22718.39000000\",\"22734.86000000\",\"235.78707000\",1658406599999,\"5362425.80850080\",8664,\"129.20321000\",\"2938592.50360720\",\"0\"],[1658406600000,\"22737.89000000\",\"22825.69000000\",\"22712.74000000\",\"22812.42000000\",\"711.05683000\",1658406779999,\"16198474.95800110\",16301,\"394.02824000\",\"8977246.34660210\",\"0\"],[1658406780000,\"22812.42000000\",\"22834.46000000\",\"22780.00000000\",\"22795.43000000\",\"403.83690000\",1658406959999,\"9208449.44244150\",10617,\"228.34091000\",\"5207166.38586460\",\"0\"],[1658406960000,\"22795.43000000\",\"22825.35000000\",\"22761.51000000\",\"22791.97000000\",\"456.48906000\",1658407139999,\"10402122.51364740\",11035,\"187.48354000\",\"4272875.42177680\",\"0\"],[1658407140000,\"22788.98000000\",\"22829.99000000\",\"22782.61000000\",\"22802.20000000\",\"354.90027000\",1658407319999,\"8093169.59332950\",10557,\"185.98408000\",\"4241191.93093150\",\"0\"],[1658407320000,\"22799.98000000\",\"22850.00000000\",\"22796.05000000\",\"22840.02000000\",\"626.20633000\",1658407499999,\"14294536.36280900\",12283,\"347.60654000\",\"7936173.22972810\",\"0\"],[1658407500000,\"22841.91000000\",\"22842.91000000\",\"22801.61000000\",\"22809.64000000\",\"546.40662000\",1658407679999,\"12469061.44992840\",11317,\"231.88685000\",\"5292036.28320190\",\"0\"],[1658407680000,\"22806.72000000\",\"22826.04000000\",\"22788.37000000\",\"22815.04000000\",\"271.34909000\",1658407859999,\"6188842.99713640\",8488,\"129.19426000\",\"2946852.75832520\",\"0\"],[1658407860000,\"22817.07000000\",\"22818.84000000\",\"22740.30000000\",\"22757.31000000\",\"326.39296000\",1658408039999,\"7435246.49132400\",9630,\"127.91284000\",\"2914037.42487180\",\"0\"],[1658408040000,\"22757.31000000\",\"22768.69000000\",\"22714.43000000\",\"22741.22000000\",\"372.33622000\",1658408219999,\"8466254.87480370\",9967,\"174.02652000\",\"3956979.66792430\",\"0\"],[1658408220000,\"22741.22000000\",\"22808.96000000\",\"22736.51000000\",\"22800.20000000\",\"476.50629000\",1658408399999,\"10856927.38240940\",10284,\"256.81013000\",\"5851988.30722570\",\"0\"],[1658408400000,\"22802.82000000\",\"22812.77000000\",\"22770.48000000\",\"22775.58000000\",\"284.37698000\",1658408579999,\"6481185.23163830\",8823,\"135.20992000\",\"3081627.81087880\",\"0\"],[1658408580000,\"22773.18000000\",\"22788.10000000\",\"22729.29000000\",\"22737.19000000\",\"383.34375000\",1658408759999,\"8722139.31207190\",10332,\"189.12384000\",\"4303258.48219330\",\"0\"],[1658408760000,\"22739.90000000\",\"22744.70000000\",\"22678.00000000\",\"22691.08000000\",\"585.64241000\",1658408939999,\"13300012.87049230\",12033,\"276.61007000\",\"6282351.95952030\",\"0\"],[1658408940000,\"22693.00000000\",\"22743.60000000\",\"22685.50000000\",\"22691.22000000\",\"404.66211000\",1658409119999,\"9188911.04992080\",10828,\"191.40822000\",\"4346731.73910020\",\"0\"],[1658409120000,\"22691.22000000\",\"22711.33000000\",\"22656.50000000\",\"22678.27000000\",\"445.21528000\",1658409299999,\"10100391.88352270\",10896,\"254.23196000\",\"5768062.72099410\",\"0\"],[1658409300000,\"22678.27000000\",\"22714.63000000\",\"22665.75000000\",\"22711.78000000\",\"421.76802000\",1658409479999,\"9570007.64489570\",11304,\"220.14795000\",\"4995463.85892930\",\"0\"],[1658409480000,\"22714.63000000\",\"22714.83000000\",\"22615.00000000\",\"22644.26000000\",\"453.34370000\",1658409659999,\"10275369.71457650\",11533,\"166.18450000\",\"3766586.31021540\",\"0\"],[1658409660000,\"22644.26000000\",\"22719.20000000\",\"22640.00000000\",\"22711.12000000\",\"374.62764000\",1658409839999,\"8498332.74689750\",10621,\"213.35017000\",\"4839905.48129550\",\"0\"],[1658409840000,\"22708.74000000\",\"22730.00000000\",\"22695.05000000\",\"22711.86000000\",\"269.14210000\",1658410019999,\"6112123.57426850\",7516,\"158.72841000\",\"3604930.15523690\",\"0\"],[1658410020000,\"22710.74000000\",\"22714.91000000\",\"22668.31000000\",\"22700.76000000\",\"261.83054000\",1658410199999,\"5942065.96726170\",7951,\"117.17214000\",\"2659381.18848430\",\"0\"],[1658410200000,\"22700.80000000\",\"22809.59000000\",\"22661.19000000\",\"22787.42000000\",\"981.70923000\",1658410379999,\"22308489.08630620\",20557,\"548.41908000\",\"12464910.77013480\",\"0\"],[1658410380000,\"22787.42000000\",\"22804.19000000\",\"22570.00000000\",\"22575.79000000\",\"963.88515000\",1658410559999,\"21855764.00668320\",21029,\"397.25595000\",\"9007945.46403650\",\"0\"],[1658410560000,\"22575.79000000\",\"22713.29000000\",\"22561.27000000\",\"22651.65000000\",\"818.68379000\",1658410739999,\"18532207.41030360\",19312,\"466.27395000\",\"10554782.92849450\",\"0\"],[1658410740000,\"22651.65000000\",\"22745.66000000\",\"22642.26000000\",\"22739.71000000\",\"559.91307000\",1658410919999,\"12705927.27690230\",14600,\"290.76463000\",\"6598876.69084030\",\"0\"],[1658410920000,\"22744.73000000\",\"22744.73000000\",\"22630.58000000\",\"22635.59000000\",\"563.83586000\",1658411099999,\"12791101.05627540\",14194,\"217.14763000\",\"4926609.62881280\",\"0\"],[1658411100000,\"22635.59000000\",\"22685.00000000\",\"22613.28000000\",\"22651.44000000\",\"509.56565000\",1658411279999,\"11539411.19920950\",13383,\"258.65135000\",\"5858080.57665780\",\"0\"],[1658411280000,\"22647.51000000\",\"22699.63000000\",\"22614.00000000\",\"22660.00000000\",\"816.02516000\",1658411459999,\"18484191.67845220\",15172,\"474.37317000\",\"10745263.71849560\",\"0\"],[1658411460000,\"22660.68000000\",\"22703.06000000\",\"22618.24000000\",\"22687.29000000\",\"530.37770000\",1658411639999,\"12018775.41940880\",13448,\"278.61855000\",\"6314338.07737080\",\"0\"],[1658411640000,\"22687.30000000\",\"22755.13000000\",\"22679.03000000\",\"22702.03000000\",\"614.30929000\",1658411819999,\"13956506.39644130\",16035,\"283.26975000\",\"6437324.53689440\",\"0\"],[1658411820000,\"22700.07000000\",\"22731.98000000\",\"22684.52000000\",\"22704.96000000\",\"301.08180000\",1658411999999,\"6836649.42603060\",9311,\"141.24287000\",\"3207388.67223460\",\"0\"],[1658412000000,\"22702.30000000\",\"22761.77000000\",\"22658.49000000\",\"22672.75000000\",\"536.75277000\",1658412179999,\"12191656.97445310\",13877,\"248.87226000\",\"5653569.10684300\",\"0\"],[1658412180000,\"22669.10000000\",\"22678.25000000\",\"22584.59000000\",\"22596.93000000\",\"611.46031000\",1658412359999,\"13834128.31017570\",14769,\"259.19112000\",\"5863728.05599590\",\"0\"],[1658412360000,\"22594.18000000\",\"22638.84000000\",\"22556.01000000\",\"22601.22000000\",\"416.39756000\",1658412539999,\"9409219.67011940\",11851,\"211.90357000\",\"4788773.90788390\",\"0\"],[1658412540000,\"22600.38000000\",\"22615.93000000\",\"22518.18000000\",\"22531.00000000\",\"651.40462000\",1658412719999,\"14699356.20203760\",13618,\"357.34192000\",\"8063719.99015790\",\"0\"],[1658412720000,\"22531.00000000\",\"22559.42000000\",\"22467.28000000\",\"22520.25000000\",\"883.31375000\",1658412899999,\"19881776.94538480\",20233,\"380.45008000\",\"8563294.74187840\",\"0\"],[1658412900000,\"22517.84000000\",\"22600.99000000\",\"22513.71000000\",\"22578.49000000\",\"654.47413000\",1658413079999,\"14758706.18805550\",15206,\"374.28674000\",\"8440500.27922880\",\"0\"],[1658413080000,\"22578.49000000\",\"22645.98000000\",\"22561.78000000\",\"22588.19000000\",\"722.42369000\",1658413259999,\"16335313.18705570\",16078,\"383.38356000\",\"8669206.53980940\",\"0\"],[1658413260000,\"22588.19000000\",\"22604.28000000\",\"22546.42000000\",\"22550.28000000\",\"443.87478000\",1658413439999,\"10021167.72270100\",12709,\"206.79876000\",\"4669105.10564470\",\"0\"],[1658413440000,\"22547.44000000\",\"22570.00000000\",\"22401.00000000\",\"22443.36000000\",\"868.91456000\",1658413619999,\"19526913.26359770\",19844,\"371.22534000\",\"8342133.49631910\",\"0\"],[1658413620000,\"22439.70000000\",\"22495.36000000\",\"22410.02000000\",\"22453.64000000\",\"474.45500000\",1658413799999,\"10654541.64676840\",14259,\"238.59629000\",\"5358272.55043710\",\"0\"],[1658413800000,\"22456.40000000\",\"22479.28000000\",\"22367.90000000\",\"22375.94000000\",\"858.85297000\",1658413979999,\"19250026.35205290\",19776,\"376.29406000\",\"8434889.04855110\",\"0\"],[1658413980000,\"22375.94000000\",\"22402.19000000\",\"22341.46000000\",\"22382.38000000\",\"927.47760000\",1658414159999,\"20749814.65537260\",22131,\"467.41657000\",\"10457968.83893360\",\"0\"],[1658414160000,\"22379.04000000\",\"22503.25000000\",\"22373.74000000\",\"22457.20000000\",\"787.39492000\",1658414339999,\"17673998.27613670\",18658,\"445.96707000\",\"10010355.78124370\",\"0\"],[1658414340000,\"22457.20000000\",\"22503.69000000\",\"22427.42000000\",\"22498.41000000\",\"494.23686000\",1658414519999,\"11103732.57599430\",11993,\"266.87686000\",\"5995329.75044250\",\"0\"],[1658414520000,\"22500.27000000\",\"22518.00000000\",\"22467.39000000\",\"22494.60000000\",\"485.20268000\",1658414699999,\"10914490.32881040\",11442,\"218.30316000\",\"4911182.67043590\",\"0\"],[1658414700000,\"22494.66000000\",\"22513.48000000\",\"22464.29000000\",\"22486.56000000\",\"424.21811000\",1658414879999,\"9541031.78484290\",10492,\"205.04368000\",\"4612026.44441580\",\"0\"],[1658414880000,\"22486.56000000\",\"22510.01000000\",\"22450.00000000\",\"22499.10000000\",\"381.02856000\",1658415059999,\"8565384.98414640\",9712,\"164.80583000\",\"3705449.70938120\",\"0\"],[1658415060000,\"22499.27000000\",\"22554.89000000\",\"22495.73000000\",\"22542.50000000\",\"671.01102000\",1658415239999,\"15118627.26824920\",14241,\"324.98096000\",\"7323034.24853550\",\"0\"],[1658415240000,\"22539.26000000\",\"22567.43000000\",\"22510.14000000\",\"22549.82000000\",\"513.54789000\",1658415419999,\"11573959.58466410\",10622,\"285.59726000\",\"6436905.51085130\",\"0\"],[1658415420000,\"22549.82000000\",\"22573.24000000\",\"22538.00000000\",\"22558.20000000\",\"380.28819000\",1658415599999,\"8577453.29348700\",9306,\"179.82449000\",\"4056190.59692710\",\"0\"],[1658415600000,\"22555.31000000\",\"22608.75000000\",\"22541.95000000\",\"22599.50000000\",\"648.23919000\",1658415779999,\"14637035.41480940\",13883,\"344.25227000\",\"7773486.19674640\",\"0\"],[1658415780000,\"22599.50000000\",\"22632.81000000\",\"22562.47000000\",\"22609.99000000\",\"506.47895000\",1658415959999,\"11450572.12798100\",12283,\"255.04288000\",\"5766341.10067780\",\"0\"],[1658415960000,\"22609.46000000\",\"22610.23000000\",\"22557.64000000\",\"22573.66000000\",\"316.48930000\",1658416139999,\"7145915.79038140\",9243,\"150.38484000\",\"3395523.28653590\",\"0\"],[1658416140000,\"22570.88000000\",\"22595.45000000\",\"22541.73000000\",\"22575.61000000\",\"313.42841000\",1658416319999,\"7073376.05879600\",9000,\"167.86512000\",\"3788345.87559670\",\"0\"],[1658416320000,\"22572.53000000\",\"22579.59000000\",\"22520.17000000\",\"22576.15000000\",\"336.01118000\",1658416499999,\"7573762.79357490\",8537,\"154.97029000\",\"3493455.98644050\",\"0\"],[1658416500000,\"22572.94000000\",\"22585.55000000\",\"22530.77000000\",\"22580.27000000\",\"344.70715000\",1658416679999,\"7775859.22530260\",8872,\"182.64767000\",\"4120682.85828140\",\"0\"],[1658416680000,\"22582.78000000\",\"22622.30000000\",\"22576.52000000\",\"22580.47000000\",\"339.20124000\",1658416859999,\"7665441.23135640\",9372,\"163.83529000\",\"3702616.42459560\",\"0\"],[1658416860000,\"22580.47000000\",\"22602.74000000\",\"22540.00000000\",\"22540.00000000\",\"226.65325000\",1658417039999,\"5117589.58691010\",7264,\"124.65740000\",\"2814942.57599910\",\"0\"],[1658417040000,\"22540.00000000\",\"22583.63000000\",\"22534.65000000\",\"22579.46000000\",\"284.21149000\",1658417219999,\"6409457.03517360\",7680,\"181.79064000\",\"4099812.43149210\",\"0\"],[1658417220000,\"22576.32000000\",\"22619.75000000\",\"22565.21000000\",\"22597.31000000\",\"322.03861000\",1658417399999,\"7274966.12065890\",8670,\"153.70009000\",\"3472267.65901930\",\"0\"],[1658417400000,\"22597.31000000\",\"22627.12000000\",\"22567.08000000\",\"22604.54000000\",\"382.58311000\",1658417579999,\"8645680.77902210\",9208,\"206.41542000\",\"4665063.99991030\",\"0\"],[1658417580000,\"22604.54000000\",\"22679.24000000\",\"22595.55000000\",\"22638.65000000\",\"513.34132000\",1658417759999,\"11621224.26405850\",12727,\"295.57066000\",\"6691962.66588730\",\"0\"],[1658417760000,\"22635.43000000\",\"22649.99000000\",\"22597.74000000\",\"22602.99000000\",\"262.50853000\",1658417939999,\"5939528.41191620\",7950,\"125.85287000\",\"2847786.43192670\",\"0\"],[1658417940000,\"22602.99000000\",\"22624.55000000\",\"22578.77000000\",\"22619.52000000\",\"275.52841000\",1658418119999,\"6227668.01880770\",7878,\"124.55555000\",\"2815486.37942980\",\"0\"],[1658418120000,\"22617.11000000\",\"22635.70000000\",\"22600.95000000\",\"22617.49000000\",\"184.82517000\",1658418299999,\"4180441.29485610\",6292,\"94.03597000\",\"2127057.83857010\",\"0\"],[1658418300000,\"22617.49000000\",\"22653.75000000\",\"22612.12000000\",\"22629.62000000\",\"322.35254000\",1658418479999,\"7297467.42938650\",7880,\"164.91270000\",\"3733435.39123250\",\"0\"],[1658418480000,\"22629.62000000\",\"22638.79000000\",\"22600.37000000\",\"22615.17000000\",\"172.80806000\",1658418659999,\"3908758.64365420\",6237,\"90.38199000\",\"2044436.16816720\",\"0\"],[1658418660000,\"22613.05000000\",\"22650.00000000\",\"22611.86000000\",\"22623.67000000\",\"238.33282000\",1658418839999,\"5393969.80908340\",6668,\"124.67580000\",\"2821889.25406390\",\"0\"],[1658418840000,\"22627.51000000\",\"22671.74000000\",\"22616.16000000\",\"22654.31000000\",\"259.71153000\",1658419019999,\"5883076.03230580\",7542,\"150.86612000\",\"3417536.53642690\",\"0\"],[1658419020000,\"22654.31000000\",\"22663.53000000\",\"22629.71000000\",\"22642.34000000\",\"164.84280000\",1658419199999,\"3733229.97298510\",5261,\"68.96541000\",\"1562027.93261990\",\"0\"],[1658419200000,\"22639.37000000\",\"22750.00000000\",\"22632.72000000\",\"22748.81000000\",\"784.09697000\",1658419379999,\"17794881.78427910\",15169,\"419.31001000\",\"9516636.31999980\",\"0\"],[1658419380000,\"22748.81000000\",\"22836.33000000\",\"22705.01000000\",\"22810.81000000\",\"760.98967000\",1658419559999,\"17338112.13430760\",17596,\"424.43382000\",\"9671471.28107210\",\"0\"],[1658419560000,\"22813.35000000\",\"22864.32000000\",\"22782.14000000\",\"22836.74000000\",\"617.37825000\",1658419739999,\"14092826.28602640\",14993,\"353.31000000\",\"8066048.21934790\",\"0\"],[1658419740000,\"22836.62000000\",\"22953.60000000\",\"22817.91000000\",\"22881.14000000\",\"1152.94784000\",1658419919999,\"26382783.06593600\",21157,\"646.25903000\",\"14788465.16710490\",\"0\"],[1658419920000,\"22881.14000000\",\"22973.86000000\",\"22860.00000000\",\"22911.23000000\",\"921.13765000\",1658420099999,\"21110065.45621150\",18053,\"404.86273000\",\"9277663.37789540\",\"0\"],[1658420100000,\"22913.28000000\",\"23043.42000000\",\"22911.23000000\",\"23039.81000000\",\"949.14123000\",1658420279999,\"21805520.54177930\",21613,\"522.31050000\",\"12001011.24156010\",\"0\"],[1658420280000,\"23039.81000000\",\"23042.64000000\",\"22960.00000000\",\"22980.78000000\",\"719.70991000\",1658420459999,\"16547353.83590860\",15360,\"376.94933000\",\"8667319.98567860\",\"0\"],[1658420460000,\"22980.78000000\",\"22987.59000000\",\"22922.47000000\",\"22938.97000000\",\"583.14425000\",1658420639999,\"13386195.44152090\",11581,\"283.64175000\",\"6510668.57851360\",\"0\"],[1658420640000,\"22936.18000000\",\"22963.08000000\",\"22915.00000000\",\"22936.78000000\",\"546.96703000\",1658420819999,\"12543744.53025320\",10511,\"327.52560000\",\"7511664.82279820\",\"0\"],[1658420820000,\"22936.78000000\",\"23096.06000000\",\"22934.90000000\",\"23066.60000000\",\"969.23675000\",1658420999999,\"22327534.66869910\",21425,\"535.34567000\",\"12330940.48409770\",\"0\"],[1658421000000,\"23066.61000000\",\"23199.15000000\",\"23051.18000000\",\"23124.87000000\",\"1446.49933000\",1658421179999,\"33442449.45953860\",27109,\"711.90925000\",\"16460989.66628220\",\"0\"],[1658421180000,\"23124.87000000\",\"23129.52000000\",\"23020.19000000\",\"23025.99000000\",\"494.86210000\",1658421359999,\"11411495.01259360\",13086,\"239.16607000\",\"5515294.12999060\",\"0\"],[1658421360000,\"23025.17000000\",\"23054.41000000\",\"23000.00000000\",\"23038.48000000\",\"492.11677000\",1658421539999,\"11333033.10541270\",11793,\"298.11386000\",\"6865754.94105570\",\"0\"],[1658421540000,\"23041.18000000\",\"23050.00000000\",\"22999.70000000\",\"23029.94000000\",\"437.28207000\",1658421719999,\"10066883.01508790\",11000,\"214.33301000\",\"4934664.11730790\",\"0\"],[1658421720000,\"23028.39000000\",\"23033.00000000\",\"22944.03000000\",\"22965.79000000\",\"602.29793000\",1658421899999,\"13843812.87492930\",12341,\"265.82091000\",\"6110262.60418730\",\"0\"],[1658421900000,\"22965.79000000\",\"23038.01000000\",\"22938.23000000\",\"22998.22000000\",\"527.01384000\",1658422079999,\"12110408.28720970\",11336,\"256.04984000\",\"5883494.64830220\",\"0\"],[1658422080000,\"22998.22000000\",\"23084.51000000\",\"22991.27000000\",\"23029.94000000\",\"471.90980000\",1658422259999,\"10872042.04569030\",10268,\"236.18621000\",\"5440479.84002200\",\"0\"],[1658422260000,\"23026.77000000\",\"23053.37000000\",\"23004.68000000\",\"23009.96000000\",\"390.53183000\",1658422439999,\"8994633.99408190\",8652,\"208.20558000\",\"4795741.54519100\",\"0\"],[1658422440000,\"23012.60000000\",\"23078.14000000\",\"23009.66000000\",\"23056.12000000\",\"360.43174000\",1658422619999,\"8306525.37795690\",8285,\"215.30716000\",\"4962000.33005630\",\"0\"],[1658422620000,\"23058.36000000\",\"23068.74000000\",\"23024.41000000\",\"23034.00000000\",\"371.81567000\",1658422799999,\"8570439.75642610\",8626,\"171.28091000\",\"3948227.18382210\",\"0\"],[1658422800000,\"23031.27000000\",\"23105.00000000\",\"23024.29000000\",\"23090.32000000\",\"376.75043000\",1658422979999,\"8687028.30731450\",10026,\"202.69684000\",\"4674169.26800610\",\"0\"],[1658422980000,\"23090.32000000\",\"23177.70000000\",\"23079.00000000\",\"23173.89000000\",\"582.45458000\",1658423159999,\"13468195.76437250\",13584,\"287.23298000\",\"6642301.55096760\",\"0\"],[1658423160000,\"23173.89000000\",\"23207.94000000\",\"23086.51000000\",\"23137.20000000\",\"912.74906000\",1658423339999,\"21127796.51317880\",16775,\"516.12066000\",\"11946744.31310010\",\"0\"],[1658423340000,\"23137.18000000\",\"23140.48000000\",\"23029.75000000\",\"23053.27000000\",\"536.40919000\",1658423519999,\"12378468.42928700\",11055,\"216.16946000\",\"4988786.17359890\",\"0\"],[1658423520000,\"23053.27000000\",\"23077.03000000\",\"22982.94000000\",\"23000.91000000\",\"487.43233000\",1658423699999,\"11230819.36535760\",11051,\"207.83671000\",\"4789168.66606700\",\"0\"],[1658423700000,\"23000.91000000\",\"23107.23000000\",\"22986.04000000\",\"23096.10000000\",\"619.38015000\",1658423879999,\"14278408.83788820\",13319,\"335.12224000\",\"7727265.91261830\",\"0\"],[1658423880000,\"23100.77000000\",\"23105.54000000\",\"23042.05000000\",\"23052.70000000\",\"248.84779000\",1658424059999,\"5740394.55985290\",7596,\"95.65251000\",\"2206713.00527410\",\"0\"],[1658424060000,\"23055.03000000\",\"23070.00000000\",\"23034.02000000\",\"23036.56000000\",\"192.91004000\",1658424239999,\"4447169.05157980\",7098,\"95.08209000\",\"2192036.32788020\",\"0\"],[1658424240000,\"23036.56000000\",\"23048.34000000\",\"22956.00000000\",\"22963.43000000\",\"661.96000000\",1658424419999,\"15220872.14812360\",15795,\"331.87053000\",\"7630914.20310280\",\"0\"],[1658424420000,\"22963.43000000\",\"22977.55000000\",\"22910.00000000\",\"22929.24000000\",\"486.58367000\",1658424599999,\"11161723.23808240\",11601,\"231.82683000\",\"5318111.92374580\",\"0\"],[1658424600000,\"22926.30000000\",\"22979.84000000\",\"22864.13000000\",\"22877.28000000\",\"693.28587000\",1658424779999,\"15884279.72231910\",16153,\"324.30003000\",\"7431174.40936770\",\"0\"],[1658424780000,\"22875.03000000\",\"22888.30000000\",\"22818.00000000\",\"22855.46000000\",\"625.14925000\",1658424959999,\"14286022.54554580\",14648,\"304.87685000\",\"6967417.89902680\",\"0\"],[1658424960000,\"22855.46000000\",\"22903.76000000\",\"22854.67000000\",\"22895.56000000\",\"439.52224000\",1658425139999,\"10059069.37270150\",10786,\"199.85484000\",\"4574141.38343810\",\"0\"],[1658425140000,\"22892.39000000\",\"22925.00000000\",\"22887.90000000\",\"22919.77000000\",\"347.00895000\",1658425319999,\"7947729.12906200\",9243,\"165.29432000\",\"3786123.87152880\",\"0\"],[1658425320000,\"22922.50000000\",\"22950.00000000\",\"22894.35000000\",\"22908.81000000\",\"302.27308000\",1658425499999,\"6927983.89108970\",8144,\"147.76484000\",\"3386678.53595910\",\"0\"],[1658425500000,\"22905.58000000\",\"22918.00000000\",\"22844.31000000\",\"22855.22000000\",\"345.86901000\",1658425679999,\"7914898.83930540\",9198,\"170.87826000\",\"3910441.31792180\",\"0\"],[1658425680000,\"22855.22000000\",\"22876.81000000\",\"22806.90000000\",\"22843.66000000\",\"439.75913000\",1658425859999,\"10044083.59040320\",10731,\"216.05524000\",\"4935045.11372160\",\"0\"],[1658425860000,\"22843.66000000\",\"22860.20000000\",\"22772.05000000\",\"22820.80000000\",\"405.37020000\",1658426039999,\"9246360.20980350\",11636,\"175.79091000\",\"4009958.57505810\",\"0\"],[1658426040000,\"22819.58000000\",\"22863.94000000\",\"22815.84000000\",\"22854.53000000\",\"348.19064000\",1658426219999,\"7954194.22991280\",9117,\"204.80859000\",\"4678839.43784270\",\"0\"],[1658426220000,\"22854.53000000\",\"22865.01000000\",\"22822.00000000\",\"22852.28000000\",\"184.72215000\",1658426399999,\"4220476.25915980\",6277,\"83.83685000\",\"1915557.02978620\",\"0\"],[1658426400000,\"22852.28000000\",\"22862.28000000\",\"22830.25000000\",\"22855.93000000\",\"204.91149000\",1658426579999,\"4681271.78860310\",7375,\"101.16774000\",\"2311317.89314440\",\"0\"],[1658426580000,\"22854.01000000\",\"22914.99000000\",\"22850.33000000\",\"22903.22000000\",\"351.07294000\",1658426759999,\"8034736.09479590\",9338,\"177.92257000\",\"4071959.46472610\",\"0\"],[1658426760000,\"22903.22000000\",\"22978.86000000\",\"22893.42000000\",\"22964.37000000\",\"450.33362000\",1658426939999,\"10330023.93426990\",10603,\"238.51522000\",\"5470881.40480730\",\"0\"],[1658426940000,\"22964.84000000\",\"23005.42000000\",\"22923.52000000\",\"22953.83000000\",\"302.19585000\",1658427119999,\"6939338.87325850\",9053,\"158.92130000\",\"3649594.06060930\",\"0\"],[1658427120000,\"22953.83000000\",\"22956.41000000\",\"22913.95000000\",\"22922.37000000\",\"222.96952000\",1658427299999,\"5114811.95752560\",6380,\"96.25649000\",\"2208181.06201800\",\"0\"],[1658427300000,\"22922.37000000\",\"22955.28000000\",\"22887.83000000\",\"22932.41000000\",\"335.96760000\",1658427479999,\"7701282.65993200\",8920,\"167.37440000\",\"3836827.81005190\",\"0\"],[1658427480000,\"22932.41000000\",\"22965.00000000\",\"22924.44000000\",\"22944.15000000\",\"166.54521000\",1658427659999,\"3821238.61695900\",5895,\"88.05551000\",\"2020390.80762930\",\"0\"],[1658427660000,\"22944.15000000\",\"22963.55000000\",\"22935.00000000\",\"22943.72000000\",\"162.45524000\",1658427839999,\"3727576.69202720\",5380,\"81.85647000\",\"1878288.21237800\",\"0\"],[1658427840000,\"22943.72000000\",\"22952.66000000\",\"22861.30000000\",\"22865.75000000\",\"332.77458000\",1658428019999,\"7620755.31801410\",8243,\"150.51964000\",\"3446953.62678340\",\"0\"],[1658428020000,\"22865.75000000\",\"22923.58000000\",\"22862.08000000\",\"22918.21000000\",\"177.38764000\",1658428199999,\"4060524.90068620\",5879,\"91.25049000\",\"2088854.30026680\",\"0\"],[1658428200000,\"22915.80000000\",\"22957.46000000\",\"22877.53000000\",\"22879.99000000\",\"259.27289000\",1658428379999,\"5941691.33582150\",7925,\"110.60407000\",\"2534947.87804810\",\"0\"],[1658428380000,\"22879.99000000\",\"22882.74000000\",\"22822.23000000\",\"22851.00000000\",\"220.60221000\",1658428559999,\"5041546.36527080\",7396,\"98.68512000\",\"2255481.41871400\",\"0\"],[1658428560000,\"22853.20000000\",\"22892.77000000\",\"22837.53000000\",\"22866.41000000\",\"249.04817000\",1658428739999,\"5695401.19830620\",6970,\"138.44786000\",\"3165953.88246450\",\"0\"],[1658428740000,\"22866.94000000\",\"22884.83000000\",\"22850.34000000\",\"22882.18000000\",\"197.30576000\",1658428919999,\"4512043.89863160\",5629,\"103.25904000\",\"2361208.70735740\",\"0\"],[1658428920000,\"22879.86000000\",\"22889.90000000\",\"22818.01000000\",\"22833.96000000\",\"223.33688000\",1658429099999,\"5103723.43874210\",7221,\"102.32564000\",\"2338527.51097550\",\"0\"],[1658429100000,\"22833.96000000\",\"22896.71000000\",\"22829.80000000\",\"22887.30000000\",\"213.34811000\",1658429279999,\"4875498.89596080\",6578,\"110.96202000\",\"2535795.94873730\",\"0\"],[1658429280000,\"22889.96000000\",\"22937.07000000\",\"22885.41000000\",\"22923.08000000\",\"260.28469000\",1658429459999,\"5963246.18935550\",7456,\"136.81198000\",\"3134306.76851200\",\"0\"],[1658429460000,\"22921.52000000\",\"22925.00000000\",\"22889.13000000\",\"22905.83000000\",\"168.71618000\",1658429639999,\"3863816.72658150\",5253,\"84.91751000\",\"1944649.01447140\",\"0\"],[1658429640000,\"22903.05000000\",\"22932.62000000\",\"22897.24000000\",\"22922.21000000\",\"186.42355000\",1658429819999,\"4271688.01133240\",5861,\"93.10003000\",\"2133270.02089910\",\"0\"],[1658429820000,\"22923.23000000\",\"22937.24000000\",\"22905.10000000\",\"22928.77000000\",\"171.95560000\",1658429999999,\"3941651.54829430\",5436,\"83.34852000\",\"1910620.82283340\",\"0\"],[1658430000000,\"22932.32000000\",\"23016.62000000\",\"22916.10000000\",\"22984.42000000\",\"395.42690000\",1658430179999,\"9077862.80224990\",9764,\"225.28735000\",\"5172681.10080120\",\"0\"],[1658430180000,\"22987.20000000\",\"23055.00000000\",\"22980.00000000\",\"23053.69000000\",\"409.96891000\",1658430359999,\"9433994.86309010\",11349,\"223.64098000\",\"5147013.91592270\",\"0\"],[1658430360000,\"23055.00000000\",\"23127.94000000\",\"23032.20000000\",\"23083.06000000\",\"743.11343000\",1658430539999,\"17154151.07704430\",15614,\"439.66095000\",\"10149801.17614670\",\"0\"],[1658430540000,\"23085.30000000\",\"23100.00000000\",\"23051.00000000\",\"23072.30000000\",\"512.21482000\",1658430719999,\"11817121.99477420\",10552,\"173.04751000\",\"3992857.05214210\",\"0\"],[1658430720000,\"23075.85000000\",\"23166.33000000\",\"23063.00000000\",\"23159.21000000\",\"680.54038000\",1658430899999,\"15740046.12294830\",14126,\"407.57644000\",\"9426944.48178830\",\"0\"],[1658430900000,\"23159.21000000\",\"23178.25000000\",\"23090.61000000\",\"23101.95000000\",\"415.17154000\",1658431079999,\"9605931.46517410\",11193,\"194.79841000\",\"4507580.36900830\",\"0\"],[1658431080000,\"23099.85000000\",\"23123.75000000\",\"23075.54000000\",\"23083.06000000\",\"289.90412000\",1658431259999,\"6696574.41779460\",7870,\"135.66154000\",\"3133814.98155390\",\"0\"],[1658431260000,\"23080.40000000\",\"23105.00000000\",\"23063.17000000\",\"23075.64000000\",\"271.85726000\",1658431439999,\"6276433.45108740\",7209,\"158.71125000\",\"3664474.39475930\",\"0\"],[1658431440000,\"23075.64000000\",\"23083.73000000\",\"23021.52000000\",\"23074.31000000\",\"333.09611000\",1658431619999,\"7680206.84738320\",8284,\"152.16591000\",\"3508627.16665830\",\"0\"],[1658431620000,\"23072.24000000\",\"23082.99000000\",\"23051.32000000\",\"23056.00000000\",\"192.21992000\",1658431799999,\"4433729.42932780\",5884,\"96.20070000\",\"2218915.07159790\",\"0\"],[1658431800000,\"23056.00000000\",\"23098.90000000\",\"22967.09000000\",\"22997.68000000\",\"451.99917000\",1658431979999,\"10415337.98220660\",10361,\"200.59135000\",\"4623346.43872740\",\"0\"],[1658431980000,\"22995.36000000\",\"23017.44000000\",\"22951.76000000\",\"22973.14000000\",\"357.09928000\",1658432159999,\"8208291.20901770\",9971,\"176.94993000\",\"4067508.40277490\",\"0\"],[1658432160000,\"22975.83000000\",\"23008.30000000\",\"22962.22000000\",\"22968.43000000\",\"279.21934000\",1658432339999,\"6417755.78579330\",7809,\"118.32391000\",\"2719835.59115120\",\"0\"],[1658432340000,\"22965.56000000\",\"23005.00000000\",\"22962.24000000\",\"22998.49000000\",\"172.47803000\",1658432519999,\"3963644.04384350\",5425,\"94.91951000\",\"2181263.54331270\",\"0\"],[1658432520000,\"23000.00000000\",\"23037.20000000\",\"22984.35000000\",\"23034.05000000\",\"129.01790000\",1658432699999,\"2968448.81057250\",5321,\"75.19795000\",\"1730299.04813210\",\"0\"],[1658432700000,\"23034.05000000\",\"23109.78000000\",\"23022.45000000\",\"23078.19000000\",\"417.71724000\",1658432879999,\"9639312.42007930\",11268,\"229.76492000\",\"5301882.26563670\",\"0\"],[1658432880000,\"23078.19000000\",\"23187.21000000\",\"23074.96000000\",\"23179.16000000\",\"701.82122000\",1658433059999,\"16244815.40051510\",15094,\"352.84718000\",\"8167202.60649620\",\"0\"],[1658433060000,\"23179.16000000\",\"23181.03000000\",\"23119.38000000\",\"23168.02000000\",\"333.74312000\",1658433239999,\"7726054.49220090\",9835,\"162.22454000\",\"3755853.92140130\",\"0\"],[1658433240000,\"23164.02000000\",\"23174.09000000\",\"23140.00000000\",\"23146.70000000\",\"280.61862000\",1658433419999,\"6497641.58736970\",8475,\"141.63746000\",\"3279636.66577850\",\"0\"],[1658433420000,\"23146.70000000\",\"23200.00000000\",\"23136.20000000\",\"23194.40000000\",\"433.83674000\",1658433599999,\"10054935.46056960\",11265,\"247.00513000\",\"5725169.32651390\",\"0\"],[1658433600000,\"23194.40000000\",\"23279.89000000\",\"23170.00000000\",\"23278.49000000\",\"844.12269000\",1658433779999,\"19598067.89894880\",16502,\"503.12871000\",\"11682803.76414940\",\"0\"],[1658433780000,\"23272.99000000\",\"23308.80000000\",\"23217.87000000\",\"23244.81000000\",\"853.96345000\",1658433959999,\"19880826.15204230\",19472,\"438.17166000\",\"10201725.47840600\",\"0\"],[1658433960000,\"23244.81000000\",\"23255.05000000\",\"23159.88000000\",\"23173.43000000\",\"601.85341000\",1658434139999,\"13961955.47071510\",13476,\"272.48270000\",\"6320847.16967450\",\"0\"],[1658434140000,\"23173.43000000\",\"23249.00000000\",\"23153.43000000\",\"23179.49000000\",\"538.35977000\",1658434319999,\"12492851.48382290\",13179,\"246.03734000\",\"5709539.09140990\",\"0\"],[1658434320000,\"23181.67000000\",\"23216.99000000\",\"23168.48000000\",\"23192.73000000\",\"328.11851000\",1658434499999,\"7609197.48306220\",9653,\"184.11216000\",\"4269928.23417940\",\"0\"],[1658434500000,\"23192.73000000\",\"23199.99000000\",\"23121.09000000\",\"23130.75000000\",\"458.04398000\",1658434679999,\"10609370.87729310\",12250,\"195.29615000\",\"4523685.64312360\",\"0\"],[1658434680000,\"23130.75000000\",\"23145.85000000\",\"23090.00000000\",\"23120.55000000\",\"361.30891000\",1658434859999,\"8349966.56587740\",10280,\"183.71860000\",\"4246024.88609870\",\"0\"],[1658434860000,\"23123.79000000\",\"23160.00000000\",\"23089.97000000\",\"23102.20000000\",\"363.22217000\",1658435039999,\"8399777.25837240\",9034,\"179.46102000\",\"4149724.96401560\",\"0\"],[1658435040000,\"23102.20000000\",\"23215.70000000\",\"23095.06000000\",\"23162.81000000\",\"894.14925000\",1658435219999,\"20709120.06372130\",12049,\"399.71885000\",\"9257591.39594320\",\"0\"],[1658435220000,\"23161.04000000\",\"23170.98000000\",\"23128.39000000\",\"23133.98000000\",\"273.33770000\",1658435399999,\"6327699.56955010\",8035,\"169.27125000\",\"3918801.11077610\",\"0\"],[1658435400000,\"23136.31000000\",\"23154.91000000\",\"23097.91000000\",\"23126.37000000\",\"272.13477000\",1658435579999,\"6293248.68539540\",8399,\"134.24952000\",\"3104537.55176200\",\"0\"],[1658435580000,\"23129.14000000\",\"23192.86000000\",\"23124.88000000\",\"23184.69000000\",\"192.92991000\",1658435759999,\"4466020.76126140\",6181,\"121.98519000\",\"2823606.07426610\",\"0\"],[1658435760000,\"23187.42000000\",\"23203.48000000\",\"23150.44000000\",\"23168.47000000\",\"252.58446000\",1658435939999,\"5856375.62237920\",7391,\"119.11169000\",\"2761741.22313110\",\"0\"],[1658435940000,\"23165.08000000\",\"23232.00000000\",\"23155.92000000\",\"23201.91000000\",\"292.65706000\",1658436119999,\"6787701.75214010\",8975,\"146.94032000\",\"3408198.74707750\",\"0\"],[1658436120000,\"23201.91000000\",\"23284.86000000\",\"23190.83000000\",\"23259.07000000\",\"566.50752000\",1658436299999,\"13170809.15007630\",14557,\"274.48504000\",\"6381762.56740400\",\"0\"],[1658436300000,\"23259.07000000\",\"23282.49000000\",\"23175.38000000\",\"23206.25000000\",\"420.49383000\",1658436479999,\"9764957.49587700\",11099,\"199.36386000\",\"4630569.89335670\",\"0\"],[1658436480000,\"23206.25000000\",\"23239.35000000\",\"23191.11000000\",\"23234.74000000\",\"303.13332000\",1658436659999,\"7034819.23568360\",8088,\"150.98731000\",\"3504405.15000630\",\"0\"],[1658436660000,\"23237.03000000\",\"23248.61000000\",\"23155.00000000\",\"23170.20000000\",\"400.94785000\",1658436839999,\"9308571.59028380\",9068,\"151.26771000\",\"3512110.38145290\",\"0\"],[1658436840000,\"23166.30000000\",\"23209.99000000\",\"23103.00000000\",\"23111.64000000\",\"589.40334000\",1658437019999,\"13649453.32335560\",12722,\"212.27444000\",\"4916728.08503920\",\"0\"],[1658437020000,\"23111.64000000\",\"23148.92000000\",\"23109.10000000\",\"23136.16000000\",\"85.40682000\",1658437199999,\"1975925.32333690\",2640,\"54.39395000\",\"1258414.47655360\",\"0\"]]", 11 "error in (no error)":errorcluster) -> (4 "Klines":dbl[][](array[numeric]) format="%#.6g", 15 "error out":errorcluster)   [LabVIEW 2022 SP3]
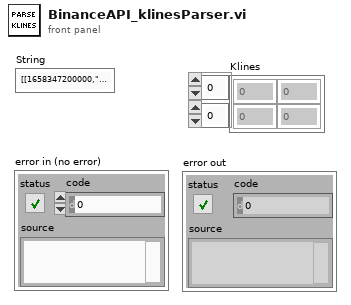
[diagram p1: front panel]
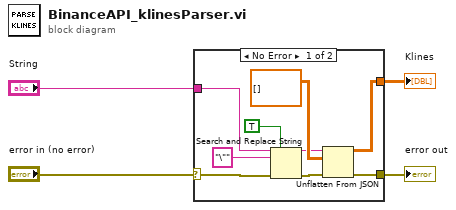
[diagram p0: block diagram]
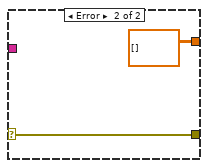
[diagram p2: hidden frame]
diagram:
  n1 = case shown="No Error" "error in (no error)" {
    selector: "error in (no error)" -> [w5 w14]
    tunnel: [w9 dbl[][] []] -> w4
    tunnel: "String" -> [w8 _]
    tunnel: [w6 w14] -> w2
    frame No Error {
      n2 = Search and Replace String(replace all?=TRUE ("replace all? (F)"), input string=w8, search string="\"", error in=w5) -> (result string=w10:string, error out=w7:errorcluster)  [unwired: 4 in, 2 out]
      n3 = Unflatten From JSON(JSON string=w10, type and defaults=dbl[][] [], error in (no error)=w7) -> (value=w9:dbl[][], error out=w6:errorcluster)  [unwired: 4 in]
    }
    frame Error {
    }
  }
  "Klines" <- w4
  "error out" <- w2
